vi "Text control 2 v6.5.vi"() -> ()   [LabVIEW 2016]
panel:
  in  "Tab Control":enum32{"Main", "Other parameters"}(tab)
  out "Line running":i32
  out "Total lines":i32
  out "Path":path=path "C:/users/rlp38/09Apr2009LTtesting/test2.txt"
  out "I vs Vg":cluster{"Y data in":dbl[], "X data in":dbl[]}[](graph)
  out "Is max":dbl format="%.2e"
  out "Id max":dbl format="%.2e"
  out "Ig max":dbl format="%.2e"
  out "Imax vs time":cluster{"Y data in":dbl[], "X data in":dbl[]}[](graph)
  out "Imin vs time":cluster{"Y data in":dbl[], "X data in":dbl[]}[](graph)
  out "I vs Vd":cluster{"Y data in":dbl[], "X data in":dbl[]}[](graph)
  in  "Script":string="#pulsedstressV d 0.03 20 0 0.5 0.0827 5\n#\n#itime m\n#gaterangemode a\n#drainrangemode a\n#pulsed on 0.05 0 0.02\n#transfer d -10 40 1 5 40 35\n#transfer d -10 40 1 5 40 35\n#transfer d -10 40 1 5 40 35\n#output d 0 40 20 0 40 1\n#\n#\n#sample 1 0.008 221 6 0.003\n#samplei 400e-6 200 6 0.002 0.1\n#vsu2pulse -10 4\n#\n#stressV 0.016 0.03 2e-4 0.1e-3 11\n#stressI 220e-7 0.08 15\n#transfer s -1 1 0.5 -0.005 0.005 0.005\n#output s 0 0 0 -0.008 0.008 0.002"
  out "Command running:":string
  out "Serial port data":string
  out "Elapsed Time":dbl caption="Elapsed Time (s)"
  in  "Time Units":u16(ring)=1 items=["Seconds", "Minutes", "Hours"]
  in  "Time Offset":dbl caption="Set Start Time (s)"
  in  "Reset":bool
  in  "Auto Reset":bool
  in  "integration time":u32(slide) max=2 step=1 scale=0.0..2.0
  out "Is on":dbl format="%.2e"
  out "Id on":dbl format="%.2e"
  out "Ig on":dbl format="%.2e"
  out "Ion vs time":cluster{"Y data in":dbl[], "X data in":dbl[]}[](graph)
  out "Ioff vs time":cluster{"Y data in":dbl[], "X data in":dbl[]}[](graph)
  out "Ig min":dbl format="%.2e"
  out "Id min":dbl format="%.2e"
  out "Is min":dbl format="%.2e"
  out "Is off":dbl format="%.2e"
  out "Id off":dbl format="%.2e"
  out "Ig off":dbl format="%.2e"
  in  "Integration time (long)":dbl=0.32 min=0.04 max=2.0 step=0.02 format="%.2f"
  in  "Integration time (short)":dbl=0.0019 min=8e-05 max=0.0019 step=8e-05 format="%^.0e"
  in  "Drain: Compliance":dbl=0.001 format="%.8f"
  in  "Gate: Compliance":dbl=0.001 format="%.8f"
  in  "Interrupt scan":bool
  in  "Interrupt program":bool
  in  "Plot output curve extrema vs time":bool
  in  "Plot transfer curve extrema vs time":bool
  in  "Gate Range\nmode":u16(ring) items=["Auto", "Limited", "Fixed"]
  in  "Gate Range":u8(slide)=6 max=11 scale=0.0..11.0
  in  "Source/Drain\nRange mode":u16(ring) items=["Auto", "Limited", "Fixed"]
  in  "Source/Drain Range":u8(slide)=6 max=11 scale=0.0..11.0
  in  "Panel Controls":T1={"Emergency Stop"=refnum, "TransGraph Max"=1e-05, "Text/Graph (text=false)"=TRUE} {"TransGraph Max" format="%.2e"}
  in  "Panel Controls 2":T2={"Emergency Stop"=refnum, "TransGraph Max"=1e-05, "Text/Graph (text=false)"=TRUE, "TransGraph Min"=1e-11} {"TransGraph Min" format="%.2e"; "TransGraph Max" format="%.2e"}
  out "error out":errorcluster
  in  "Delay before read (ms)":u32=1000
  in  "byte count":u32=64
  in  "Serial End Mode for Reads":u16(ring)=2 items=["None", "LastBit", "TermChar"]
  in  "Timeout (ms)":u32=10000
  in  "Enable Termination\nChar (T)":bool=TRUE
  in  "Termination char\n(0xA = '\\n' = LF)\n(0xD = '\\r' = CR)":u8=13 format="%.0x"
  in  "flow control":u16(ring) items=["None"=0, "XON/XOFF"=1, "RTS/CTS"=2, "DTR/DSR"=4]
  in  "stop bits":u16(ring)=10 items=["1.0"=10, "1.5"=15, "2.0"=20]
  in  "parity":u16(ring) items=["None", "Odd", "Even", "Mark", "Space"]
  in  "data bits":u16=8 min=5 max=8 step=1
  in  "VISA resource name":refnum<visa-resource-name>="COM6"
  in  "baud rate":u32=9600
  out "Timings Indicator":T3
  in  "Timings (overwritten by the Front Panel)":T4={"integration time"=0, "Short/Long integration time"=0.00064, "hold time (sec)"=0.0, "delay time (sec)"=0.0, "Step Time (0 disables)"=0.0, "sweep method"=0, "Pulse period"=0.005, "Base voltage"=0.0, "Pulse width"=0.0005} {"Pulse width" min=0.0005 max=0.1 step=0.0001 format="%.4f"; "Base voltage" format="%^.4e"; "Pulse period" min=0.005 max=1.0 step=0.0001 format="%.4f"; "sweep method" items=["Continuous", "Pulsed"]; "Step Time (0 disables)" format="%.2f"; "delay time (sec)" format="%.4f"; "hold time (sec)" format="%.4f"; "Short/Long integration time" format="%^.0e"; "integration time" scale=0.0..2.0}
  in  "SMU4":cluster{"on/off":bool, "Voltage":dbl} {"Voltage" min=-100.0 max=100.0 format="%.2f"}
  in  "Full Reset":bool
  in  "Standby":T5
  out "SMU4 Indicator":cluster{"on/off":bool, "Voltage":dbl} {"Voltage" min=-100.0 max=100.0 format="%.2f"}
  in  "Gate":T6={"Gate Start"=0.0, "Gate Stop"=2.0, "Gate Step (linear only)"=1.0, "Gate Compliance"=0.0001, "Gate PComp"=0.0, "Range mode"=0, "Range"=6} {"Range" max=11 scale=0.0..11.0; "Range mode" items=["Auto", "Limited", "Fixed"]; "Gate PComp" format="%^.2e"; "Gate Compliance" format="%^.2e"; "Gate Step (linear only)" format="%^.4e"; "Gate Stop" format="%^.4e"; "Gate Start" format="%^.4e"}
  in  "Drain 2":T7={"Drain Start"=0.0, "Drain Stop"=2.0, "Drain Compliance"=0.0001, "Drain Step"=1.0, "Drain PComp"=0.0, "Range mode"=0, "Range"=6} {"Range" max=11 scale=0.0..11.0; "Range mode" items=["Auto", "Limited", "Fixed"]; "Drain PComp" format="%^.2e"; "Drain Step" format="%^.4e"; "Drain Compliance" format="%^.2e"; "Drain Stop" format="%^.4e"; "Drain Start" format="%^.4e"}
  # "Time"
  # "Syntax:\nitime [s|m|l] time(sec): [s|m|l] determines the integration time setting (small|medium|long) and time sets the value.\nNOTE: The value of the integration time has to be within the range allowed by its category (s|m|l), otherwise, the closest value will be used. (e.g. if the category is set to short but the time value is very long, the actual value used will be the maximum short integration time.\nIntegration times:\n    Short: Default: 640 us. Range: 8E-5 - 1.92E-3 seconds.\n    Medium: Fixed at 1 NPL cycle (0.02 seconds).\n    Long: Default: 16 NPL cycles (0.32 seconds). Range: 2-100 NPL cycles (0.04 seconds - 2 seconds).\ngaterangemode [a|l|f]\ndrainrangemode [a|l|f]\npulsed [on|off] PulsePeriod(sec) PulseBaseVoltage PulseONWidth(sec)\nstandby [on l off]\nwait NumMilliseconds\nwait-min NumMinutes\n# texthere = comment\nSMU4 [ON|OFF] Voltage\ntransfer [s|d] VgStart VgStop VgStep VdStart VdStop VdStep\noutput [s|d] VgStart VgStop VgStep VdStart VdStop VdStep\nsample Vg Vd NumSamples Time(s) SampleInterval(s)\nsamplei Idg NumSamples Time(s) SampleInterval(s) VDGcompliance\n100 samples is approximately 13 seconds with medium integration\n# if in doubt use SampleInterval(s) = 0.004\nstressV VG VD IGcompliance IDcompliance Duration(sec)\nstressI IDG VDGcompliance Duration(sec)\nvsu2pulse Bias Duration(s)\npulsedstressV [s|d] VEstop VgON VgOFF Period(s) PulseONwidth(s) Vd\nsample-fpp Vg Vd NumSamples Time\nresample-fpp Vg Vd\ntransfer-fpp [s|d] VgStart VgStop VgStep VdStart VdStop VdStep\noutput-fpp [s|d] VgStart VgStop VgStep VdStart VdStop VdStep\nserial SerialPortCommand"
  # "1\n2\n3\n4\n5\n6\n7\n8\n9\n10\n11\n12\n13\n14\n15\n16\n17\n18\n19\n20"
  # "Serial port settings"
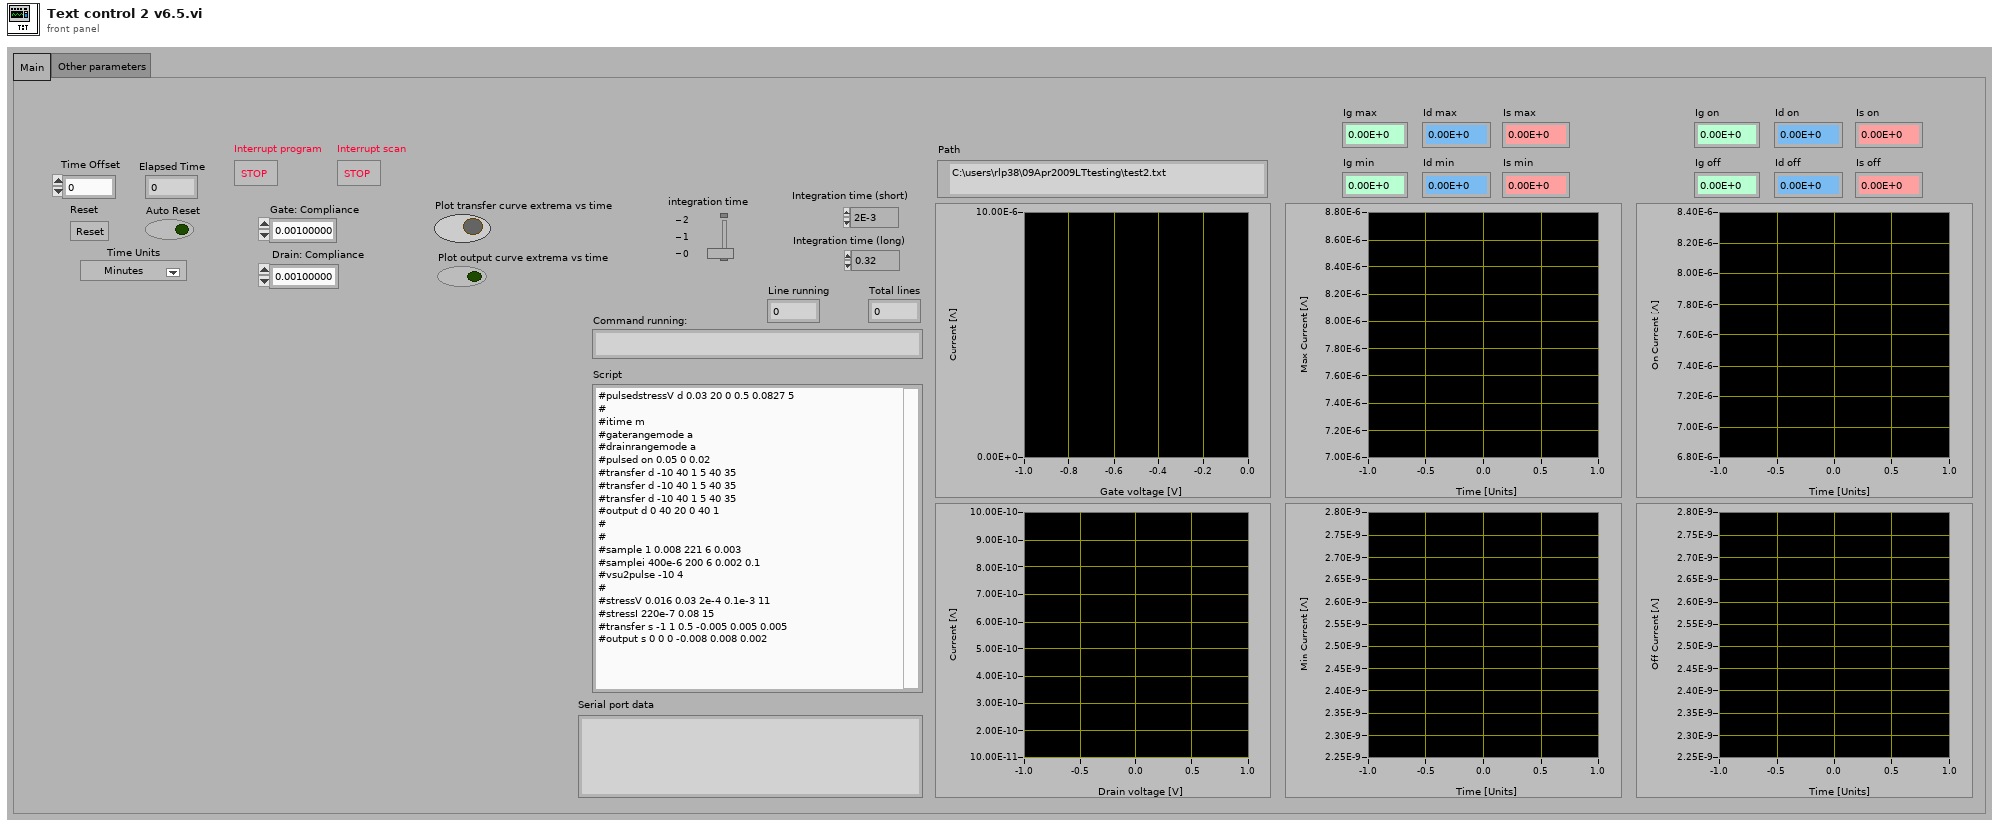
[diagram p1: front panel]
types:
  T1 = cluster{"Emergency Stop":refnum<vi>, "TransGraph Max":dbl, "Text/Graph (text=false)":bool}
  T2 = cluster{"Emergency Stop":refnum<vi>, "TransGraph Max":dbl, "Text/Graph (text=false)":bool, "TransGraph Min":dbl}
  T3 = cluster{"integration time (0:s, 1:m, 2:l)":u32, "Short/Long integration time":dbl, "hold time (sec)":dbl, "delay time (sec)":dbl, "Step Time (0 disables)":dbl, "sweep method":u16, "Pulse period":dbl, "Base voltage":dbl, "Pulse width":dbl}
  T4 = cluster{"integration time":u32, "Short/Long integration time":dbl, "hold time (sec)":dbl, "delay time (sec)":dbl, "Step Time (0 disables)":dbl, "sweep method":u16, "Pulse period":dbl, "Base voltage":dbl, "Pulse width":dbl}
  T5 = cluster{"Gate Standby":bool, "Drain Standby":bool}
  T6 = cluster{"Gate Start":dbl, "Gate Stop":dbl, "Gate Step (linear only)":dbl, "Gate Compliance":dbl, "Gate PComp":dbl, "Range mode":u16, "Range":u8}
  T7 = cluster{"Drain Start":dbl, "Drain Stop":dbl, "Drain Compliance":dbl, "Drain Step":dbl, "Drain PComp":dbl, "Range mode":u16, "Range":u8}
  T8 = enum16{"open", "replace", "create", "open or create", "replace or create", "replace or create with confirmation"}
  T9 = cluster{"V2 Start":dbl, "V2 Step":dbl, "Number of points":i32}
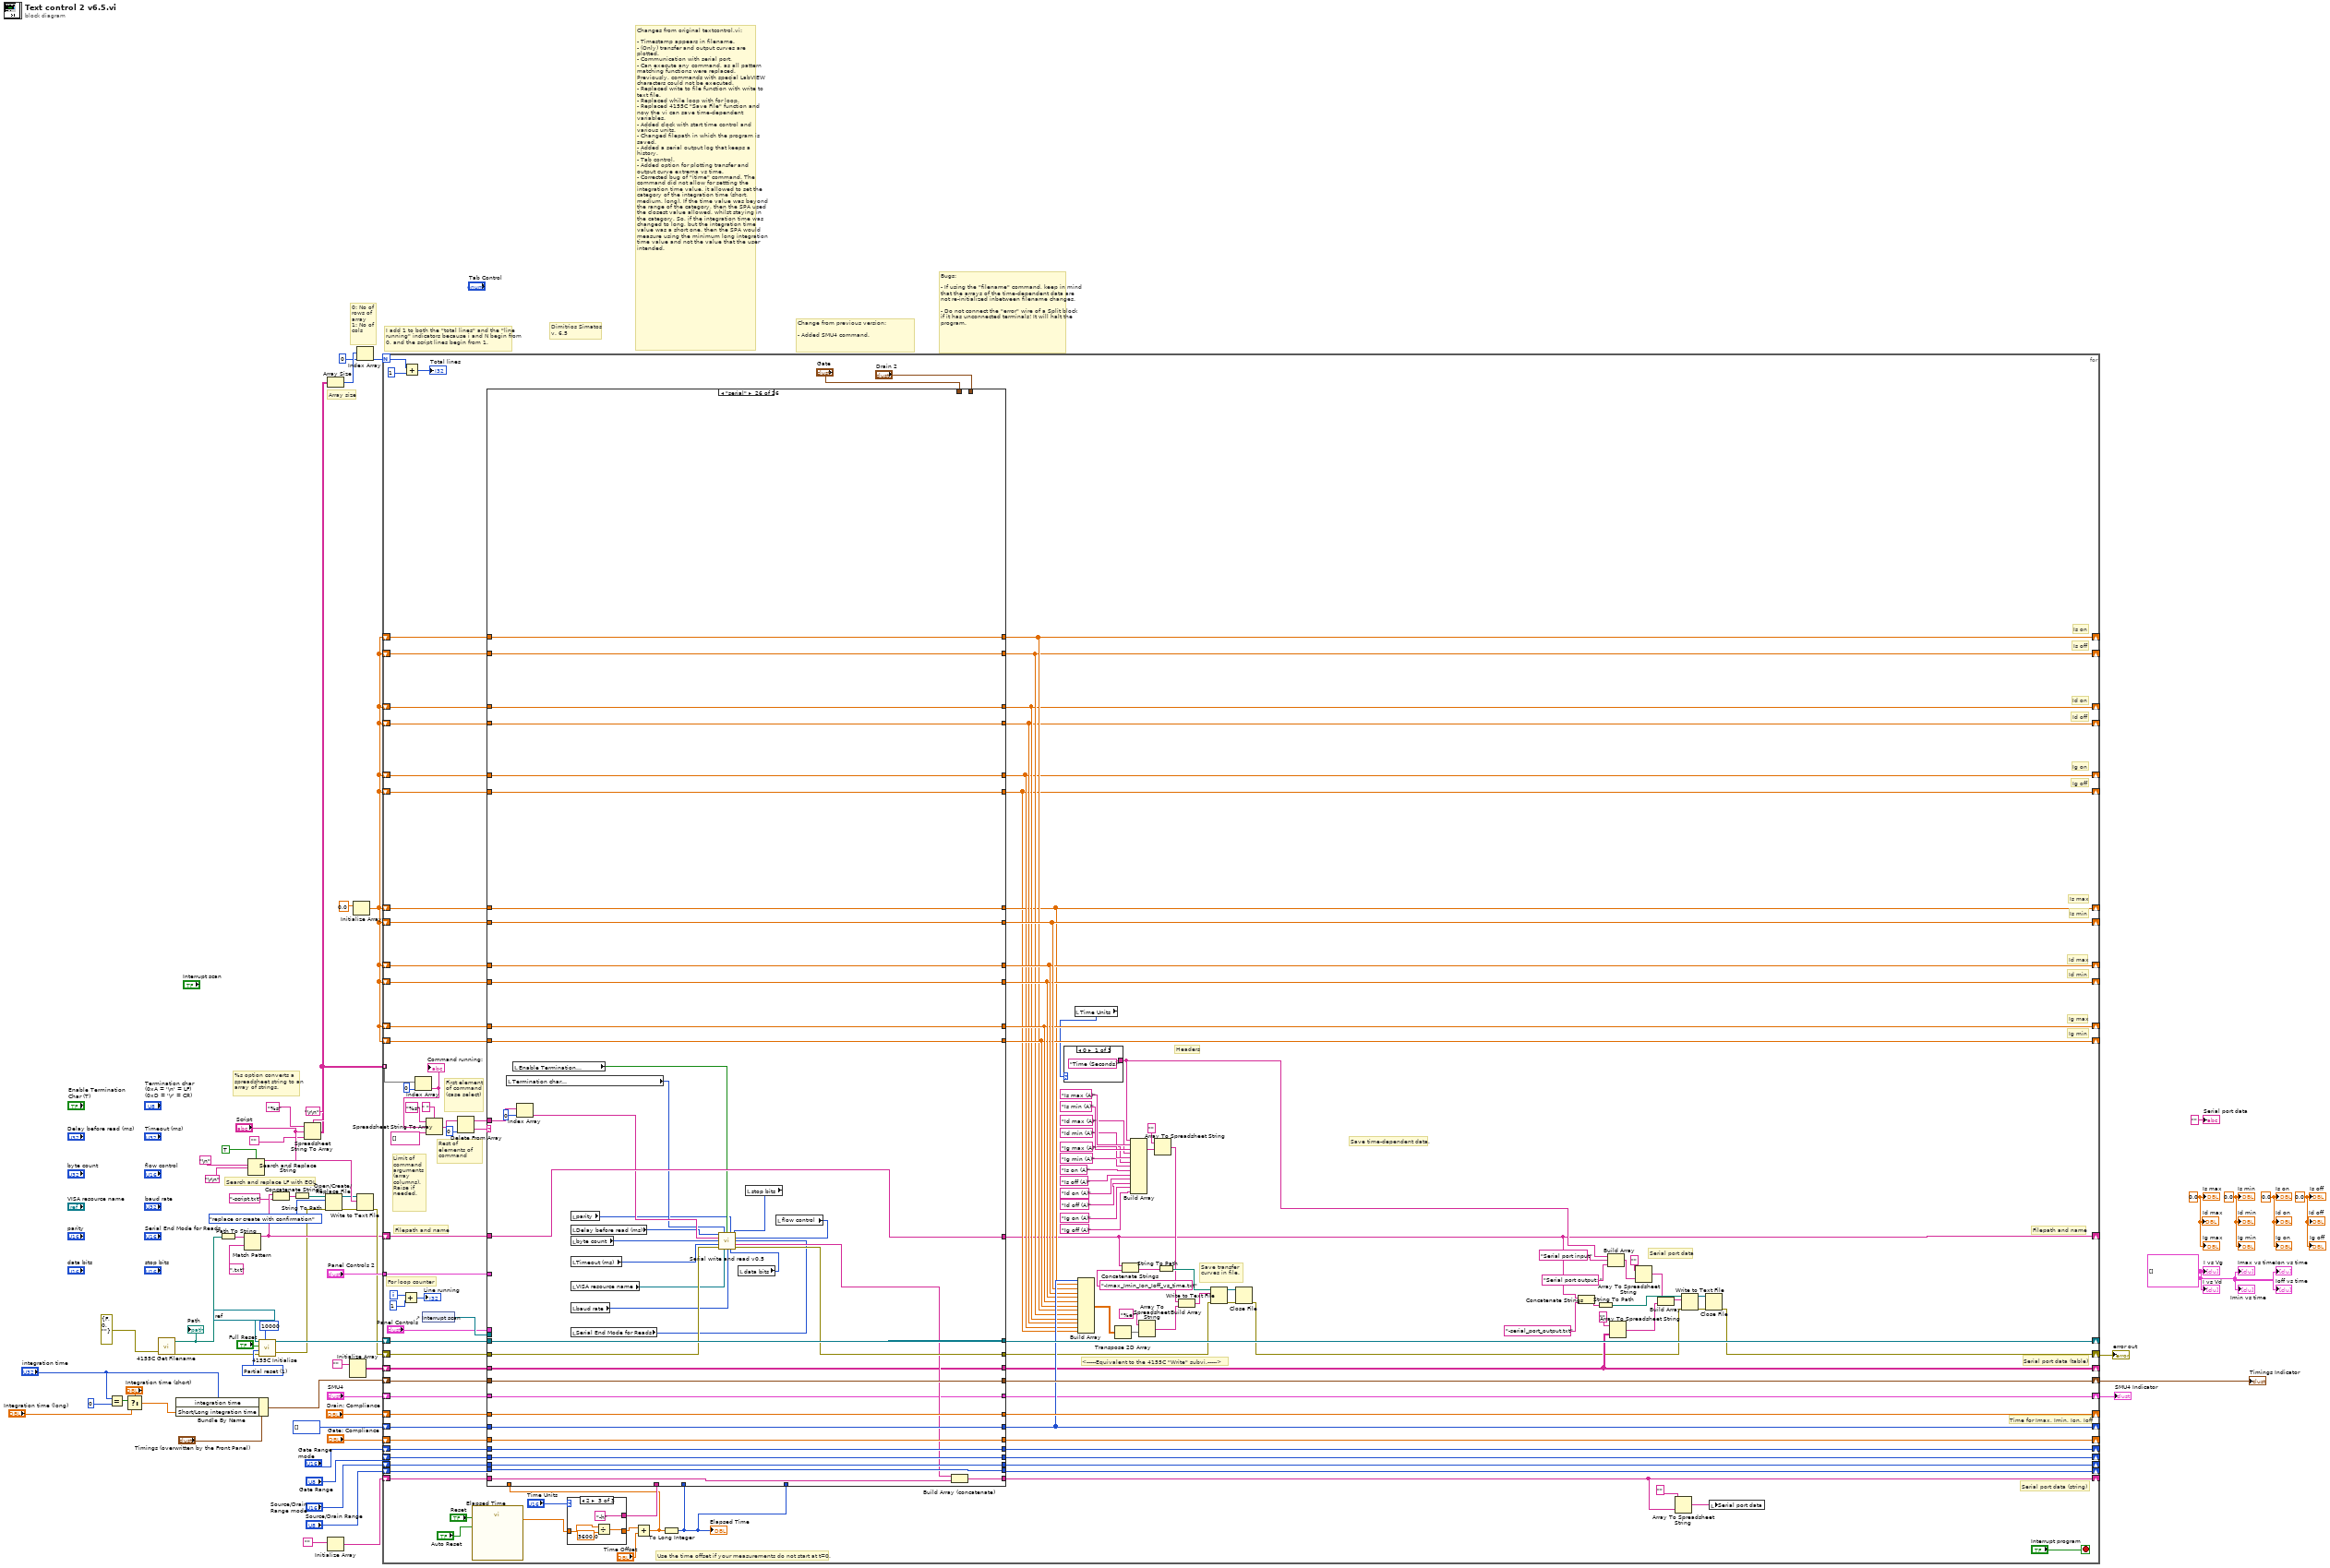
[diagram p0: block diagram]
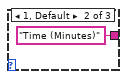
[diagram p2: hidden frame]
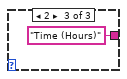
[diagram p3: hidden frame]
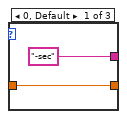
[diagram p4: hidden frame]
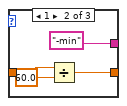
[diagram p5: hidden frame]
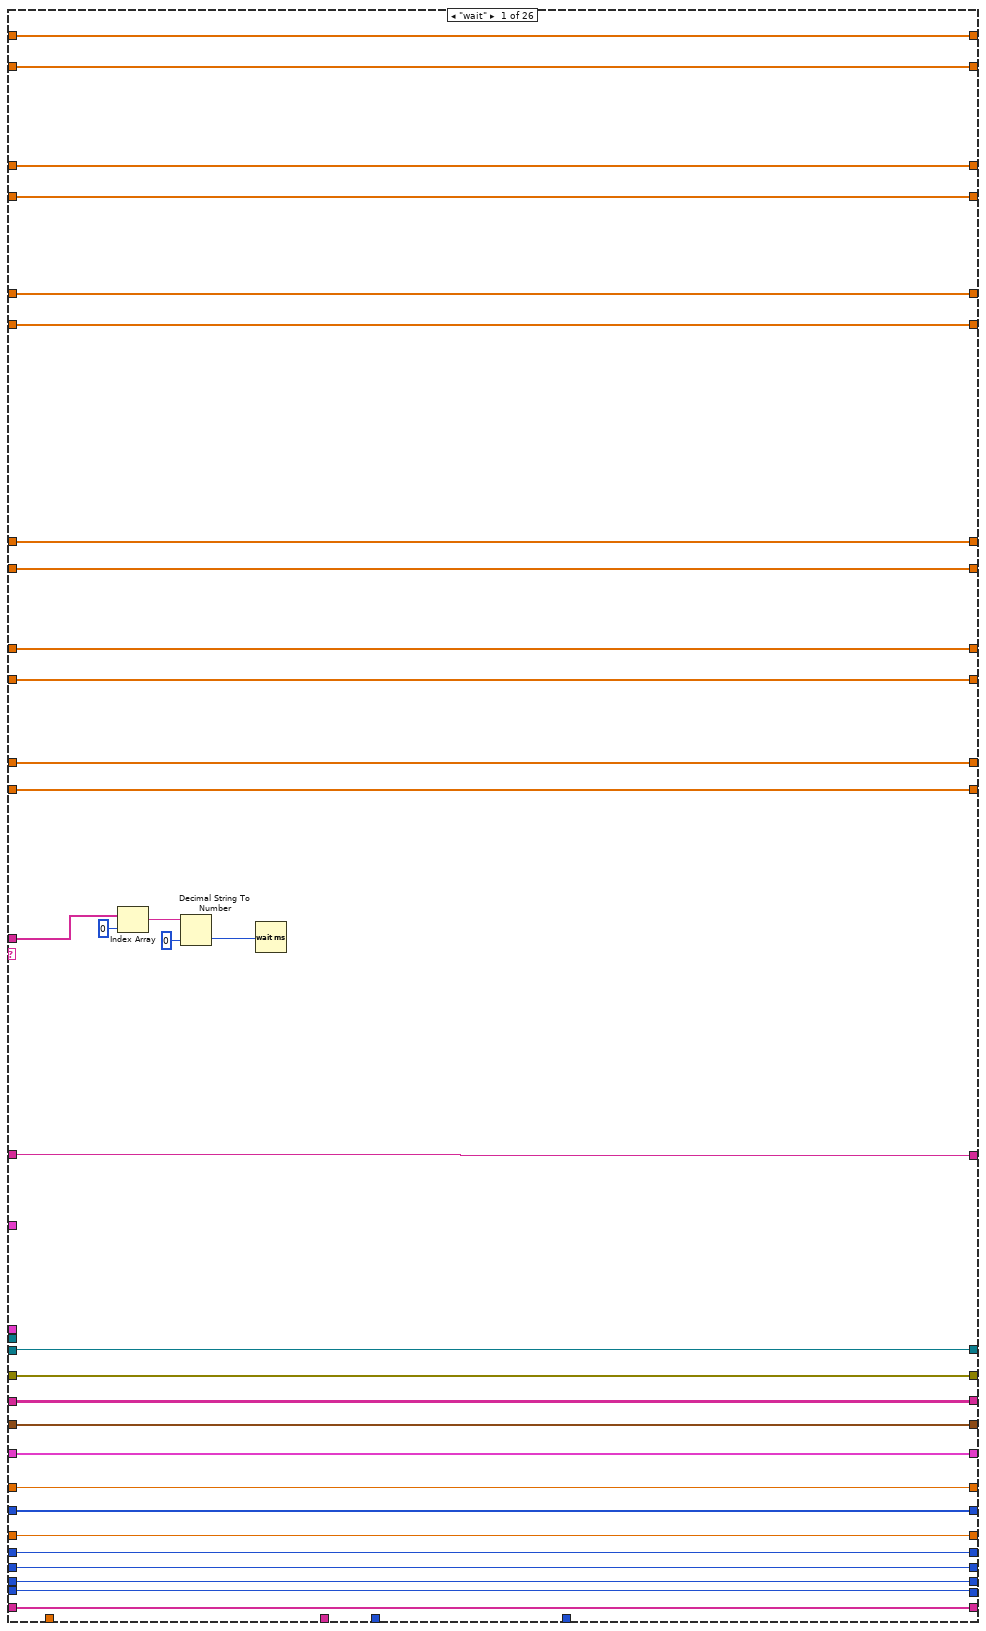
[diagram p6: hidden frame]
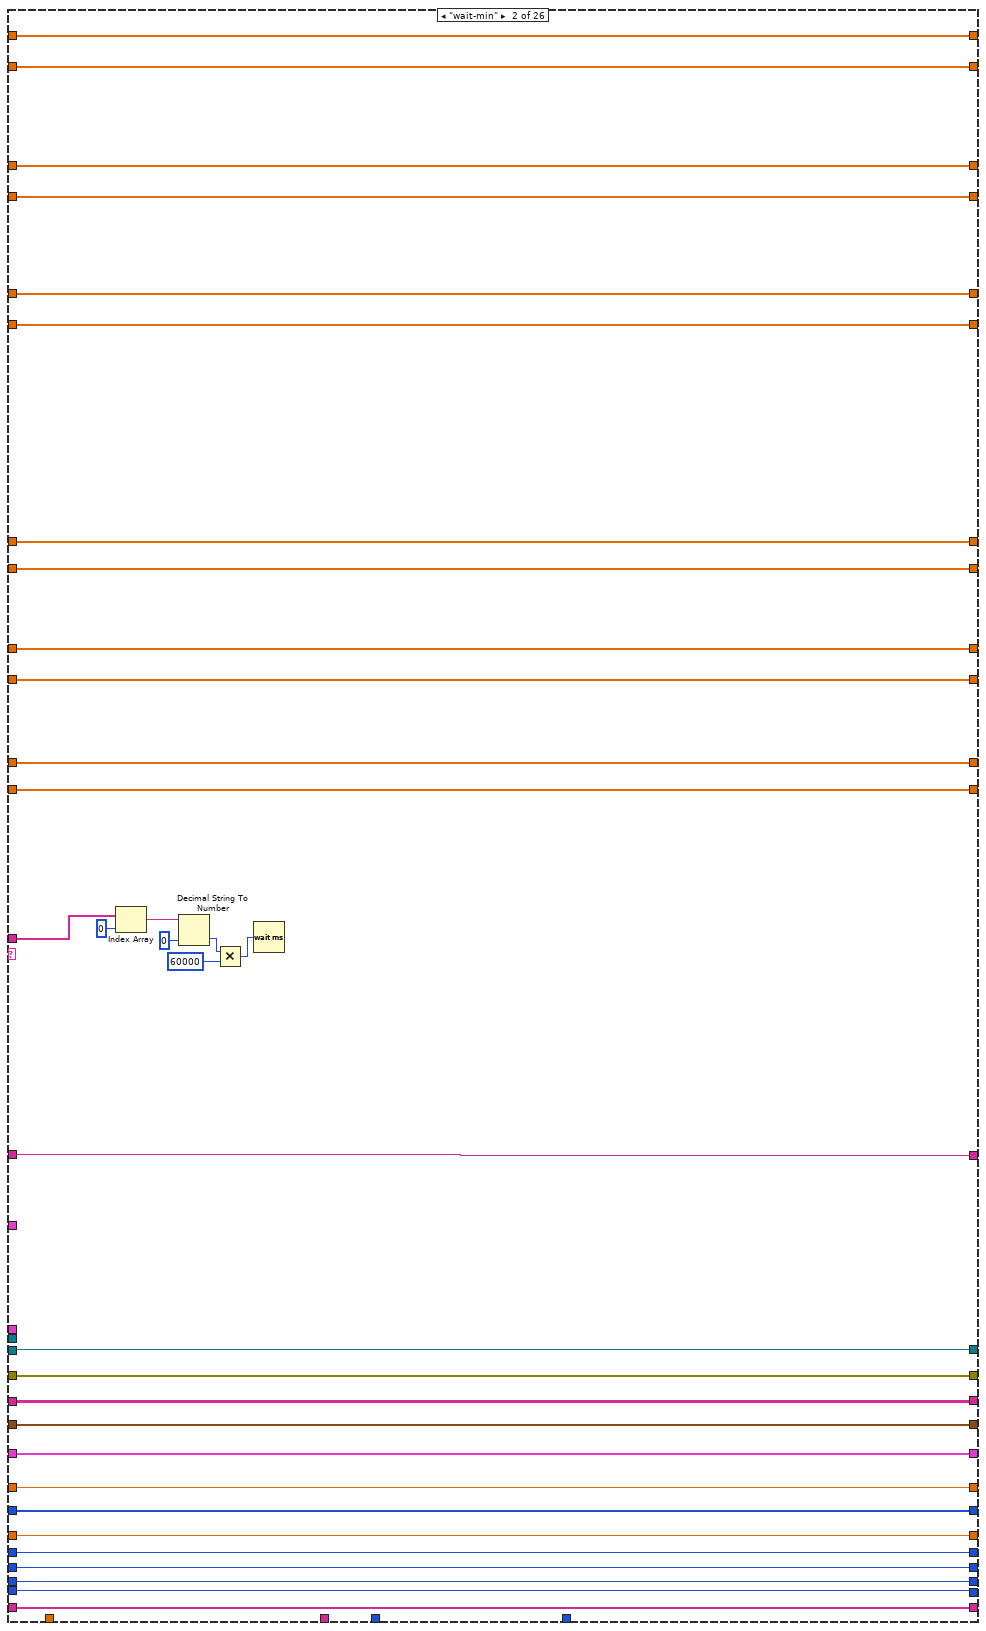
[diagram p7: hidden frame]
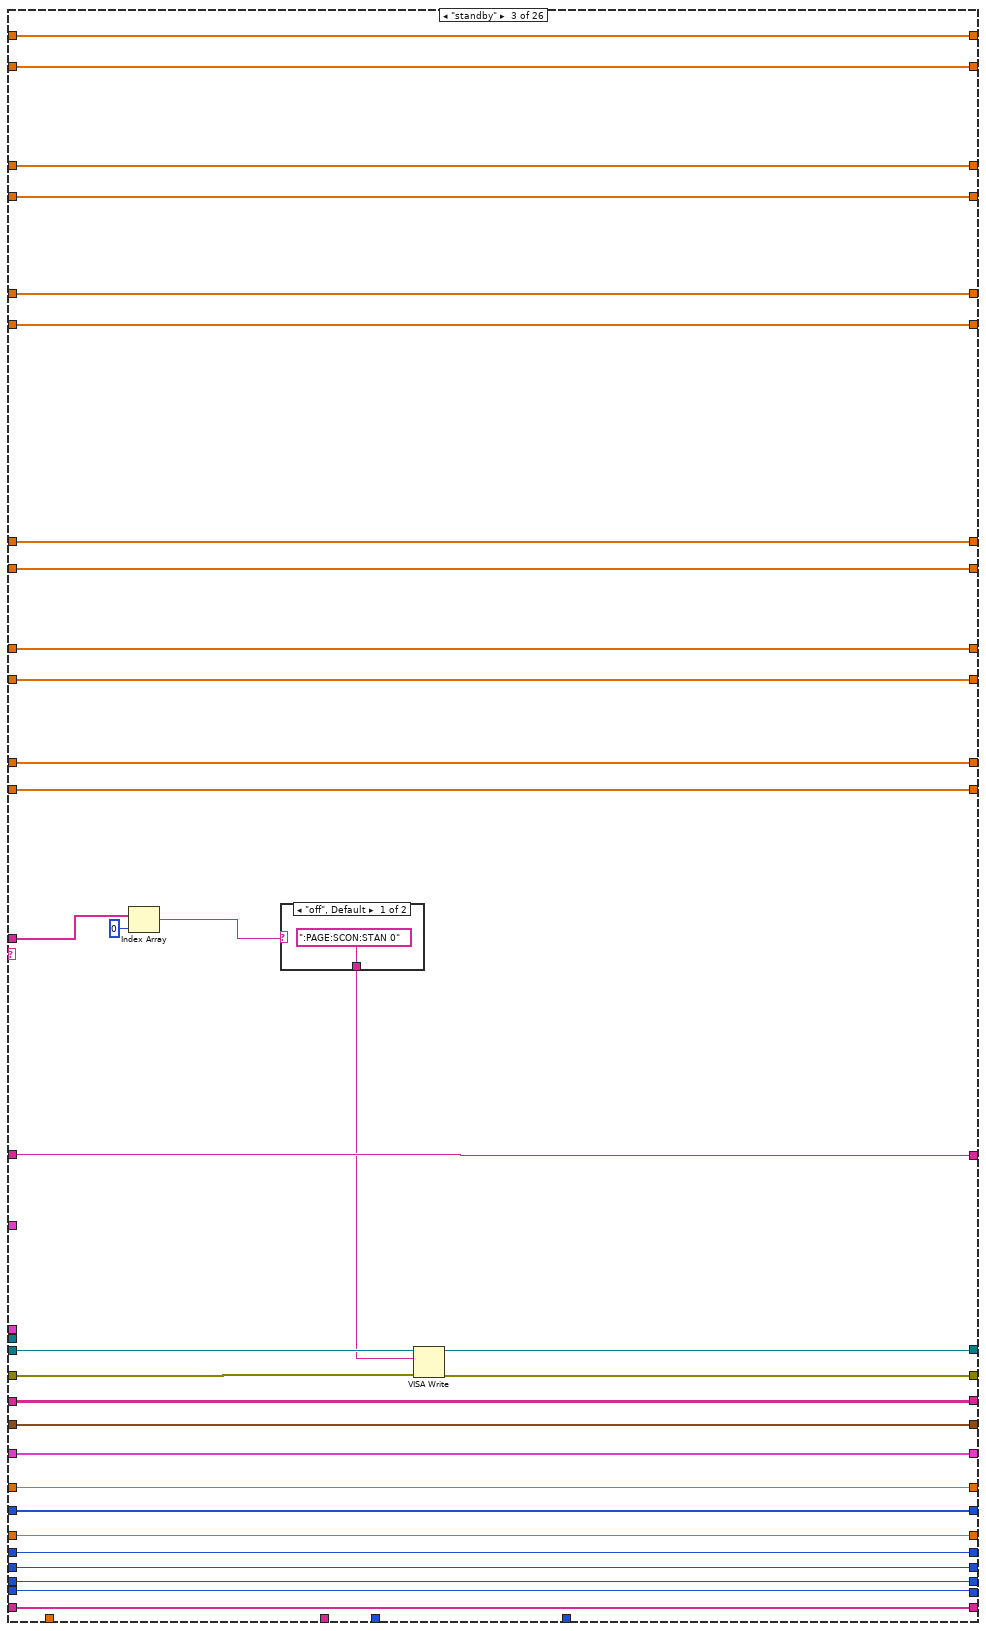
[diagram p8: hidden frame]
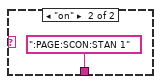
[diagram p9: hidden frame]
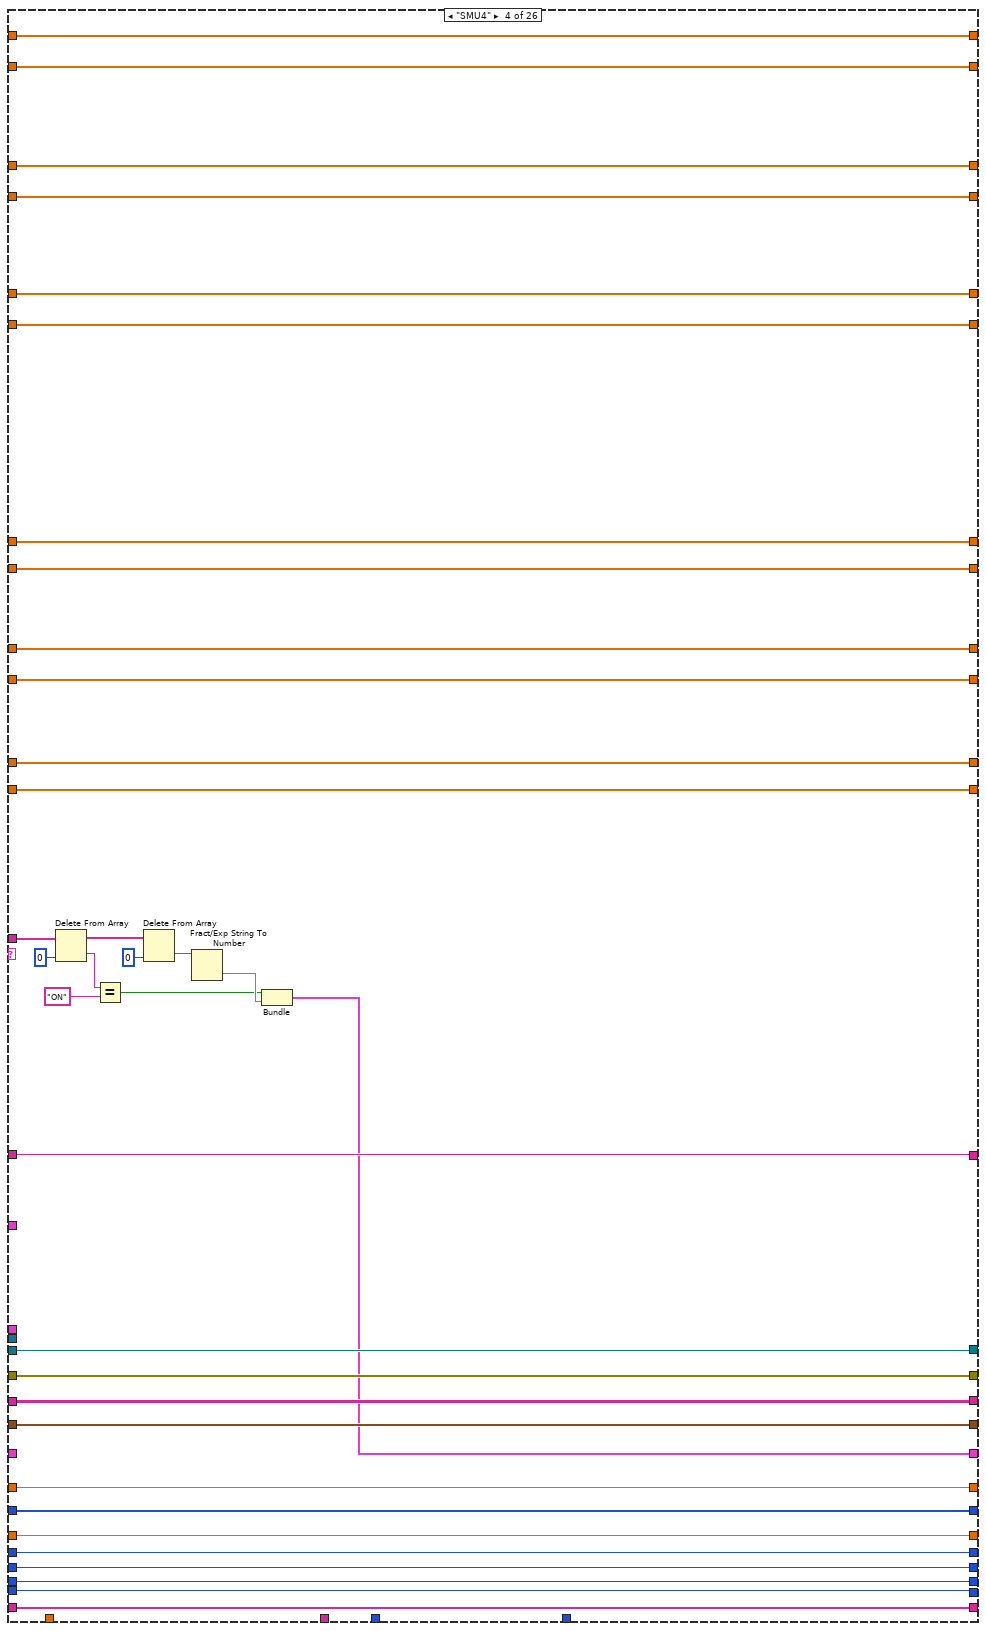
[diagram p10: hidden frame]
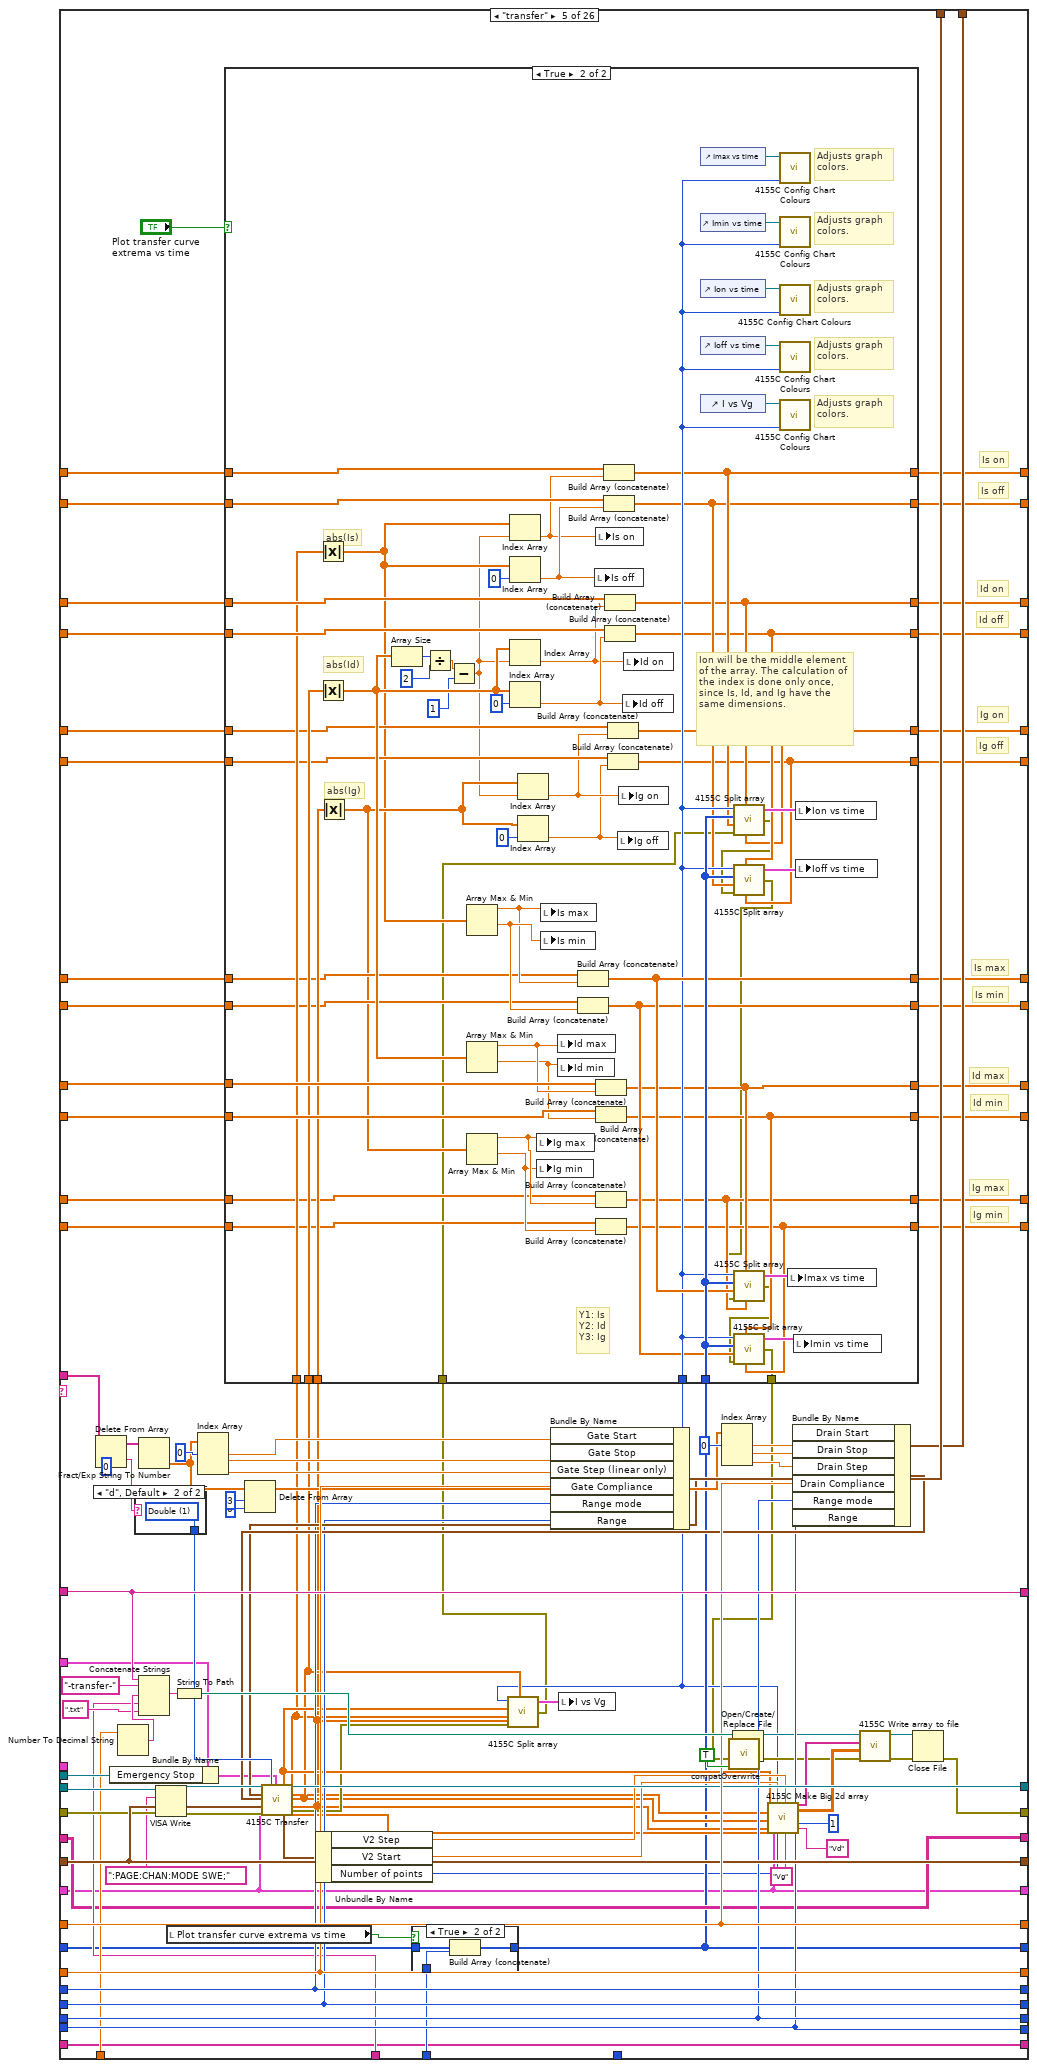
[diagram p11: hidden frame]
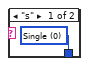
[diagram p14: hidden frame]
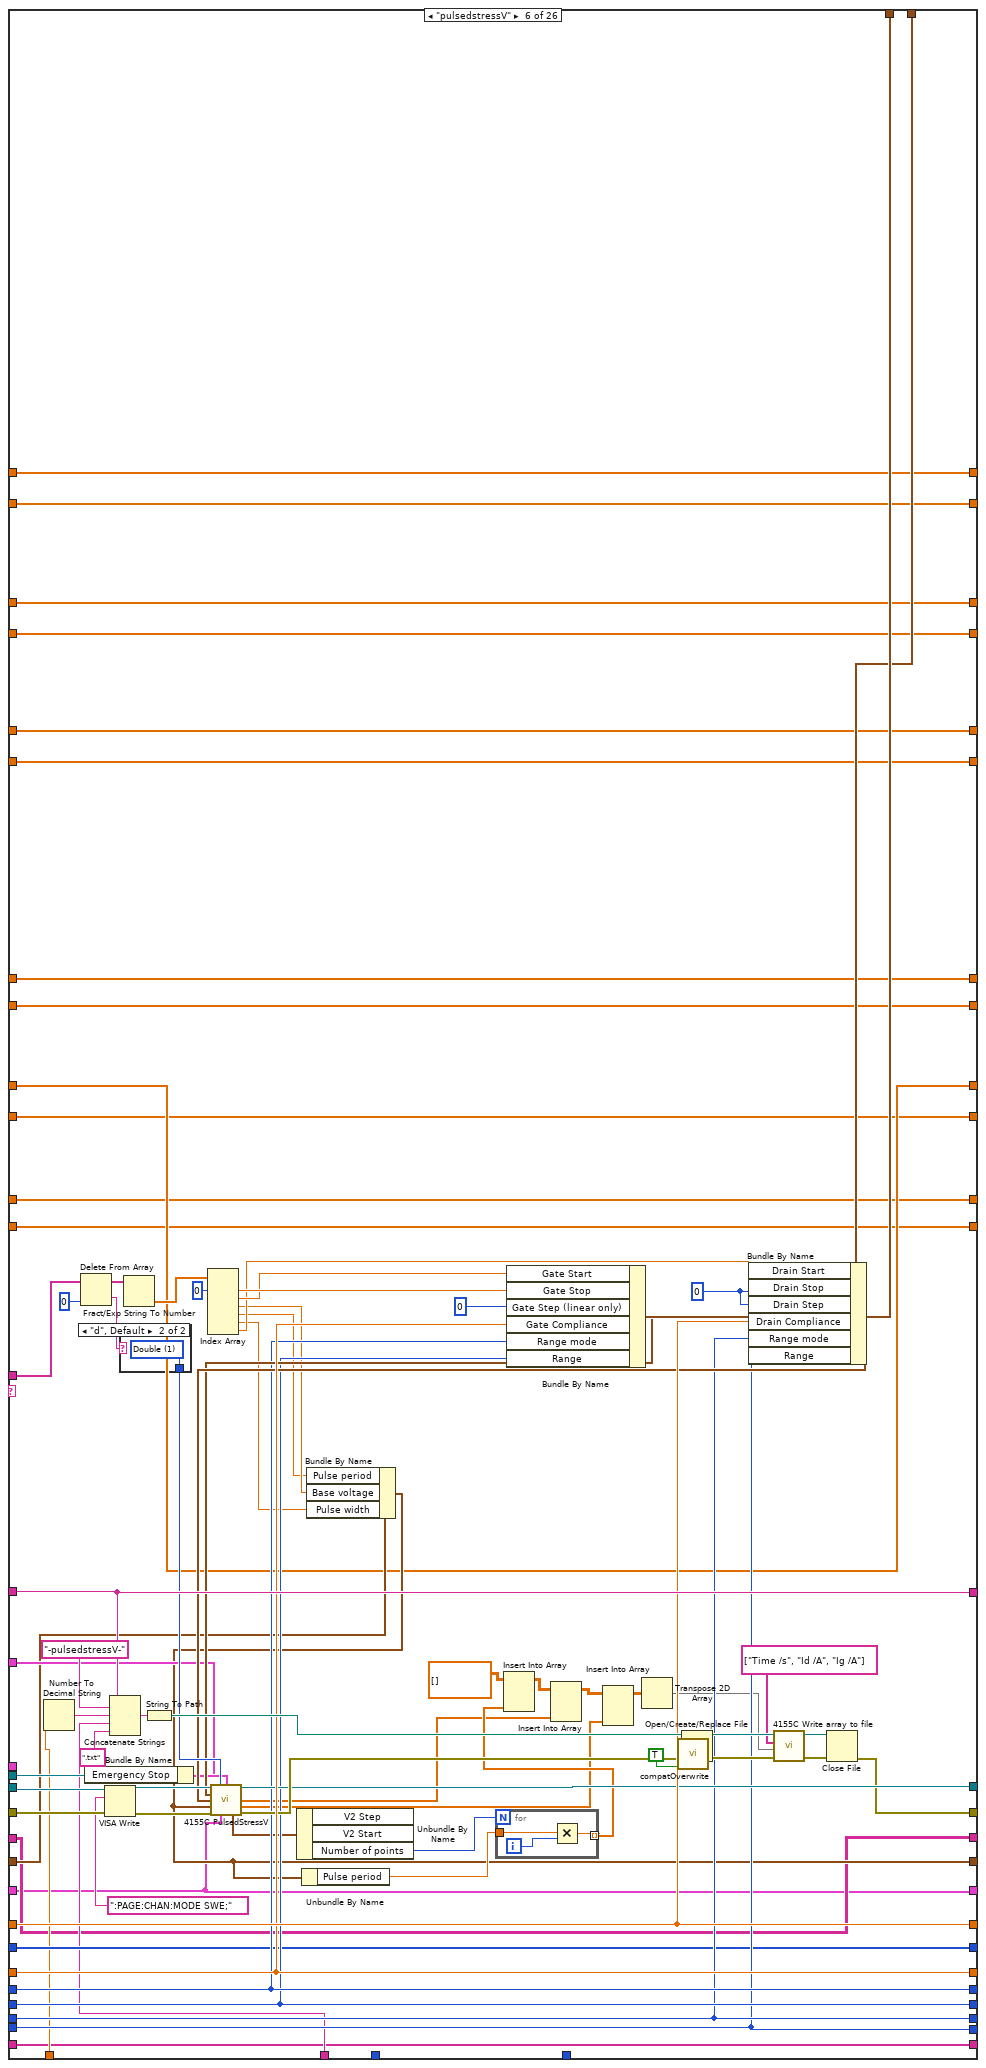
[diagram p15: hidden frame]
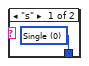
[diagram p16: hidden frame]
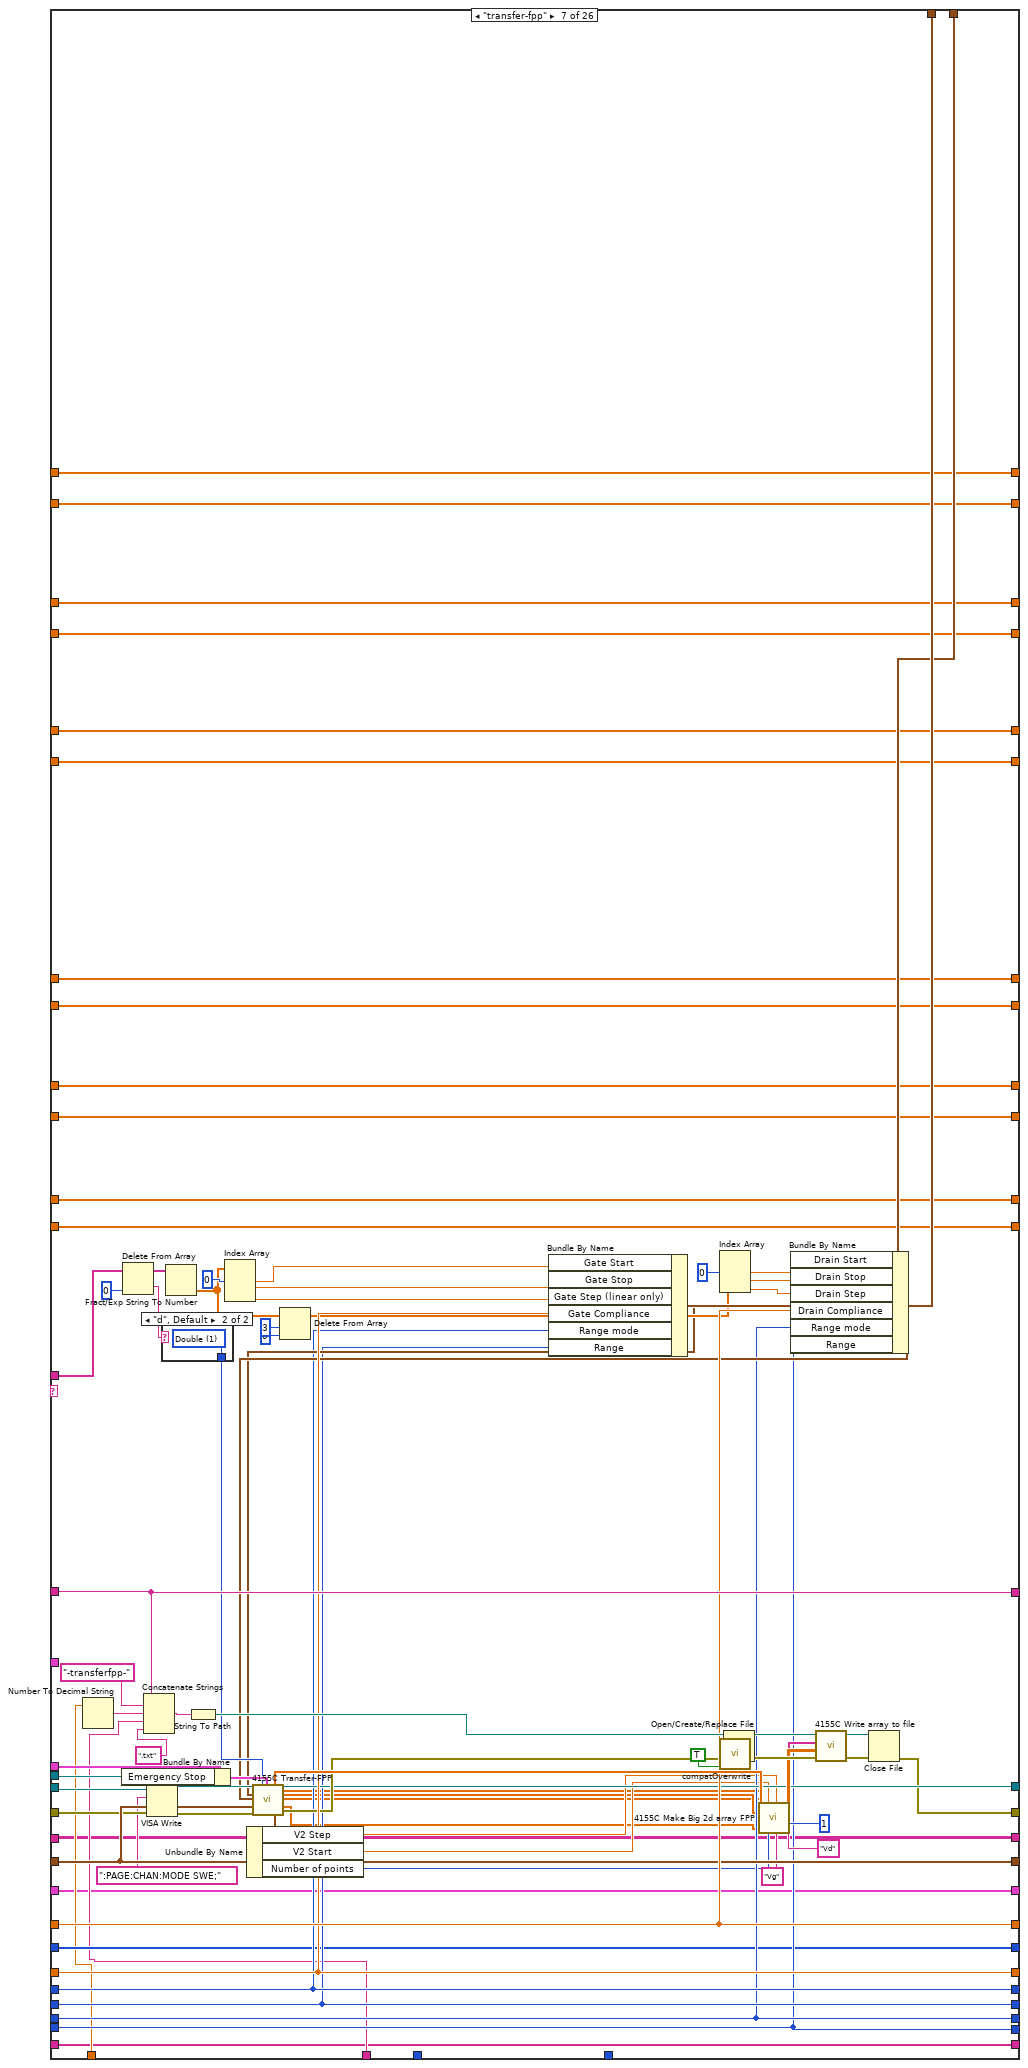
[diagram p17: hidden frame]
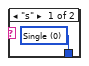
[diagram p18: hidden frame]
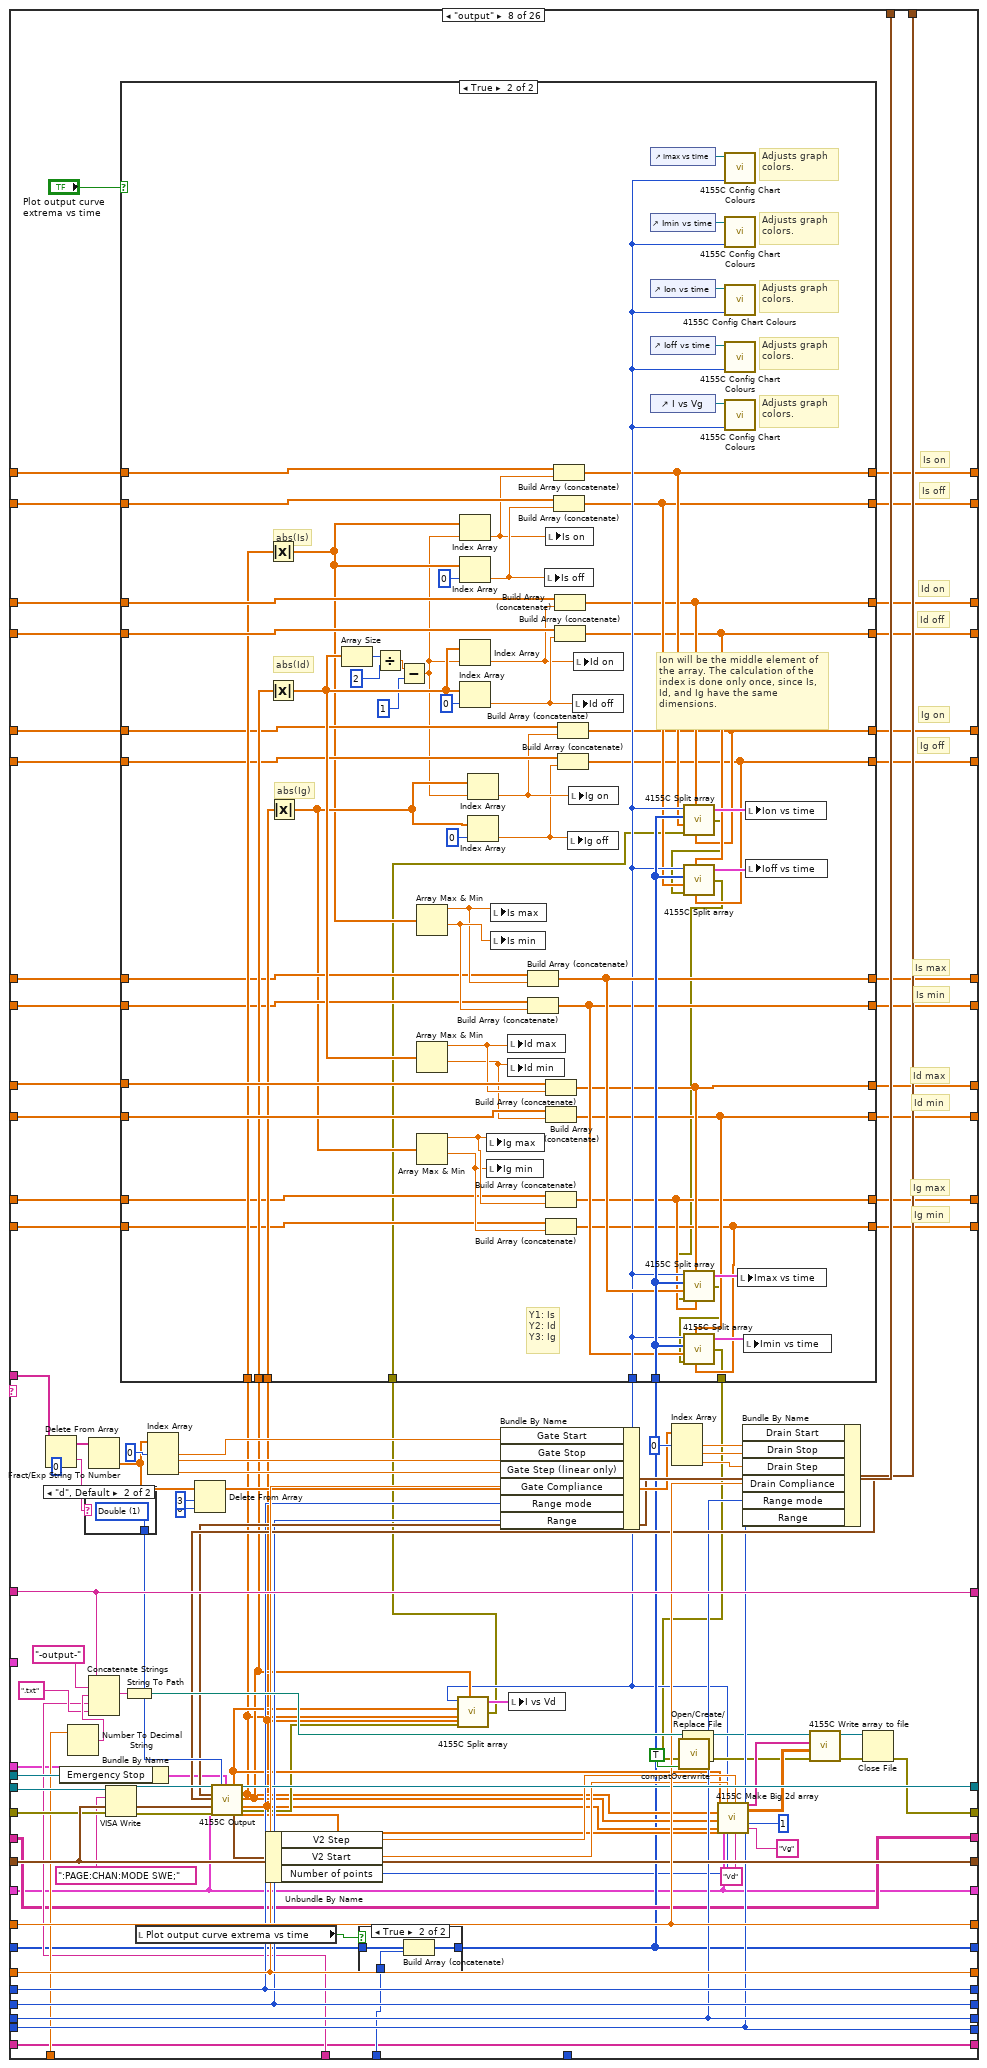
[diagram p19: hidden frame]
diagram:
  w8 = cluster{"Y data in":dbl[], "X data in":dbl[]}[] [] ("I vs Vg")
  w9 = 0.0 ("Is off")
  w10 = 0.0 ("Is on")
  w11 = 0.0 ("Is min")
  w12 = 0.0 ("Is max")
  w58 = u16 1 items=["Reset All", "Partial reset"] ("Type of reset")
  # "Change from previous version:\n\n- Added SMU4 command."
  # "I add 1 to both the \"total lines\" and the \"line running\" indicators because i and N begin from 0, and the script lines begin from 1."
  # "Bugs:\n\n- If using the \"filename\" command, keep in mind that the arrays of the time-dependent data are not re-initialized inbetween filename changes. \n\n- Do not connect the \"error\" wire of a Split block if it has unconnected terminals! It will halt the program."
  # "Array size"
  # "%s option converts a spreadsheet string to an array of strings."
  # "0: No of rows of array\n1: No of cols"
  # "Dimitrios Simatos\nv. 6.5"
  # "Changes from original textcontrol.vi:\n\n- Timestamp appears in filename.\n- (Only) transfer and output curves are plotted.\n- Communication with serial port.\n- Can execute any command, as all pattern matching functions were replaced. Previously, commands with special LabVIEW characters could not be executed.\n- Replaced write to file function with write to text file.\n- Replaced while loop with for loop.\n- Replaced 4155C \"Save File\" function and now the vi can save time-dependent variables.\n- Added clock with start time control and various units.\n- Changed filepath in which the program is saved.\n- Added a serial output log that keeps a history.\n- Tab control.\n- Added option for plotting transfer and output curve extrema vs time.\n- Corrected bug of \"itime\" command. The command did not allow for settting the integration time value, it allowed to set the category of the integration time (short, medium, long). If the time value was beyond the range of the category, then the SPA used the closest value allowed, whilst staying in the category. So, if the integration time was changed to long, but the integration time value was a short one, then the SPA would measure using the minimum long integration time value and not the value that the user intended."
  # "Search and replace LF with EOL"
  n1 = Equal?(x="integration time", y=u32 0) -> (x = y?=w59:bool)
  n2 = Select(t="Integration time (short)", s=w59, f="Integration time (long)") -> (s? t:f=w17:dbl)
  n3 = call "4155C Get Filename.vi"("error in (no error)"=errorcluster {"status"=FALSE, "code"=0, "source"=""}) -> ("error out"=w53:errorcluster, "path"=w28:path)  [unwired: 2 in, 1 out]
  "Path" <- w28
  n4 = Bundle By Name(cluster="Timings (overwritten by the Front Panel)", "integration time"="integration time", "Short/Long integration time"=w17) -> (w51:T4)
  n5 = Path To String(path=w28) -> (string=w29:string)
  n6 = Match Pattern(string=w29, regular expression=".txt") -> (before substring=w15:string)  [unwired: 1 in, 3 out]
  n7 = Search and Replace String(replace all?=TRUE ("replace all? (F)"), input string="Script", search string="\n", replace string="\r\n") -> (result string=w41:string)  [unwired: 4 in, 3 out]
  n8 = call "4155C Initialise.vi"("VISA resource name in"=refnum<visa-resource-name> "GPIB0::14::INSTR", "Reset"="Full Reset", "Type of reset"=w58, "error in (no error)"=w53, "VISA Timeout Value"=u32 10000) -> ("VISA Resource Name out"=w52:refnum<visa-resource-name>, "error out"=w6:errorcluster)
  n9 = Concatenate Strings(w15, "-script.txt" ("string")) -> (w16:string)
  n10 = String To Path(string=w16) -> (path=w4:path)
  n11 = Spreadsheet String To Array(delimiter (Tab)="\r\n", format string="%s", spreadsheet string="Script", array type (2D Dbl)="") -> (array=w32:string[][])
  n12 = Open/Create/Replace File(file path (use dialog)=w4, error in=w6, operation (0:open)=T8."replace or create with confirmation") -> (refnum out=w3:refnum<file>, error out=w5:errorcluster)  [unwired: 3 in, 1 out]
  n13 = Array Size(array=w32) -> (size(s)=w36:i32[])
  n14 = Initialize Array("") -> (w21:string[])  [unwired: 1 in]
  n15 = Initialize Array("") -> (w19:string[][])  [unwired: 2 in]
  n16 = Initialize Array(0.0 ("element")) -> (w23:dbl[])  [unwired: 1 in]
  n17 = Index Array(array=w36, index=0) -> (element=w34:i32)
  n18 = Write to Text File(file (use dialog)=w3, text=w41, error in=w5) -> (error out=w25:errorcluster)  [unwired: 1 in, 2 out]
  n19 = for {
    N: w34 -> [w132]
    shift-left: "Source/Drain Range" -> [w173]
    shift-right: [w169] -> _
    shift-left: "Source/Drain\nRange mode" -> [w174]
    shift-right: [w170] -> _
    shift-left: "Gate Range" -> [w175]
    shift-right: [w171] -> _
    shift-left: "Gate Range\nmode" -> [w176]
    shift-right: [w172] -> _
    shift-left: "Gate: Compliance" -> [w185]
    shift-right: [w181] -> _
    shift-left: "Drain: Compliance" -> [w186]
    shift-right: [w182] -> _
    shift-left: w51 -> [w187]
    shift-right: [w183] -> w18
    shift-left: w25 -> [w188]
    shift-right: [w68] -> w27
    shift-left: w52 -> [w189]
    shift-right: [w184] -> _
    shift-left: w15 -> [w190]
    shift-right: [w71] -> _
    tunnel: "Panel Controls 2" -> [w167]
    shift-right: [w83] -> _
    shift-left: w23 -> [w166]
    shift-right: [w119] -> _
    shift-left: i32[] [] -> [w162]
    tunnel: w32 -> [w161] mode=indexing
    shift-right: [w82] -> _
    shift-left: w23 -> [w138]
    shift-right: [w113] -> _
    shift-left: w21 -> [w124]
    shift-right: [w114] -> _
    shift-left: w19 -> [w116]
    shift-right: [w76] -> _
    shift-left: w23 -> [w104]
    shift-right: [w77] -> _
    shift-left: w23 -> [w103]
    shift-right: [w81] -> _
    shift-left: w23 -> [w92]
    shift-right: [w80] -> _
    shift-left: w23 -> [w91]
    shift-right: [w74] -> _
    shift-left: w23 -> [w90]
    shift-right: [w84] -> _
    shift-left: w23 -> [w89]
    shift-right: [w75] -> _
    shift-left: w23 -> [w88]
    shift-right: [w73] -> _
    shift-left: w23 -> [w87]
    shift-right: [w79] -> _
    shift-left: w23 -> [w86]
    shift-right: [w78] -> _
    shift-left: w23 -> [w85]
    shift-right: [w64] -> w1
    shift-left: "SMU4" -> [w168]
    i -> [w127]
    stop <- "Interrupt program" stop-if-true
    # "Is off"
    # "Is on"
    # "Ig off"
    # "Ig on"
    # "Is min"
    # "Is max"
    # "Ig min"
    # "Ig max"
    # "Id min"
    # "Id max"
    # "Id off"
    # "Id on"
    # "Filepath and name"
    # "Limit of command arguments (array columns). Raise if needed."
    # "Serial port data (string)"
    # "Serial port data (table)"
    # "Serial port data"
    # "For loop counter"
    # "<-----Equivalent to the 4155C \"Write\" subvi.----->"
    # "Headers"
    # "Save transfer curves in file."
    # "Filepath and name"
    # "Save time-dependent data."
    # "Use the time offset if your measurements do not start at t=0."
    # "Time for Imax, Imin, Ion, Ioff"
    # "Rest of elements of command"
    # "First element of command\n(case select)"
    n20 = Add(x=w127, y=1) -> (x+y=→"Line running":i32)
    n21 = Add(x=w132, y=1) -> (x+y=→"Total lines":i32)
    n22 = Index Array(array=w161, index=0 ("line index")) -> (element=w156:string)
    "Command running:" <- w156
    n23 = control-ref of="Interrupt scan"() -> (w180:refnum<vi>)
    n24 = Spreadsheet String To Array(delimiter (Tab)=" ", format string="%s", spreadsheet string=w156, array type (2D Dbl)=string[] []) -> (array=w154:string[])
    n25 = Delete From Array(array=w154, index=0) -> (deleted portion=w105:string, array with subset deleted=w153:string[])  [unwired: 1 in]
    n26 = call "Elapsed Time"("Reset"="Reset", "Auto Reset"="Auto Reset") -> ("Elapsed Time (s)"=w163:dbl)  [unwired: 10 in, 7 out]
    n27 = case shown="2" "Time Units" {
      tunnel: ["-sec" "-min" "-h"] -> w164
      tunnel: [w194 w198 w201] -> w134
      tunnel: w163 -> [w194 w197 w202]
      frame 0, Default {
      }
      frame 1 {
        n28 = Divide(x=w197, y=60.0) -> (x/y=w198:dbl)
      }
      frame 2 {
        n29 = Divide(x=w202, y=3600.0) -> (x/y=w201:dbl)
      }
    }
    n30 = Add(x=w134, y="Time Offset") -> (x+y=w133:dbl)
    n31 = To Long Integer(number=w133) -> (32bit integer=w118:i32)
    "Elapsed Time" <- w118
    n32 = case shown="\"serial\"" w105 {
      tunnel: w153 -> [w234 w267 w299 w311 w428 w535 w670 w785 w941 w969 w1038 w1079 w1118 w1153 w1181 _ _ w1327 w1402 _ w1495 w1553 w1609 w1693 w1769 w1803]
      tunnel: w190 -> [w229 w263 w297 w324 w435 w594 w678 w792 w949 w986 w1027 w1071 w1111 w1147 w1174 w1207 w1263 w1305 w1384 w1429 w1482 w1540 w1597 w1687 w1765 w1805]
      tunnel: w189 -> [w228 w262 w288 w323 w406 w579 w647 w763 w917 w987 w1028 w1072 w1112 w1148 w1175 w1212 w1265 w1333 w1408 w1433 w1501 w1559 w1615 w1699 w1723 w1809]
      tunnel: w188 -> [w227 w261 w287 w322 w405 w578 w646 w762 w914 w988 w1029 w1073 w1113 w1149 w1176 w1211 w1236 w1332 w1407 w1432 w1500 w1558 w1614 w1698 w1722 w1808]
      tunnel: w187 -> [w226 w260 w296 w320 w431 w555 w674 w788 w945 w996 w1037 w1070 w1110 w1146 w1173 w1210 w1260 w1296 w1376 w1438 w1475 w1533 w1590 w1686 w1764 w1810]
      tunnel: w186 -> [w225 w259 w295 w319 w433 w592 w676 w790 w947 w995 w1036 w1078 w1117 w1152 w1180 w1209 w1245 w1331 w1406 w1441 w1499 w1557 w1613 w1697 w1773 w1811]
      tunnel: w185 -> [w224 w258 w294 w317 w432 w591 w675 w789 w946 w994 w1035 w1077 w1116 w1151 w1179 w1208 w1246 w1306 w1385 w1440 w1483 w1541 w1598 w1688 w1766 w1813]
      tunnel: [w228 w262 w286 w323 w430 w589 w672 w787 w943 w987 w1028 w1072 w1112 w1148 w1175 w1212 w1265 w1297 w1358 w1431 w1476 w1534 w1591 w1639 w1725 w1809] -> w184
      tunnel: [w227 w261 w285 w322 w429 w588 w671 w786 w942 w988 w1029 w1073 w1113 w1149 w1176 w1211 w1235 w1307 w1359 w1430 w1484 w1542 w1599 w1638 w1724 w1807] -> w117
      tunnel: [w226 w260 w296 w320 w431 w551 w674 w788 w945 w989 w1030 w1070 w1110 w1146 w1173 w1210 w1260 w1296 w1376 w1438 w1475 w1533 w1590 w1686 w1764 w1810] -> w183
      tunnel: [w225 w259 w295 w319 w433 w592 w676 w790 w947 w995 w1036 w1078 w1117 w1152 w1180 w1209 w1245 w1331 w1406 w1441 w1499 w1557 w1613 w1697 w1773 w1811] -> w182
      tunnel: [w224 w258 w294 w317 w432 w591 w675 w789 w946 w994 w1035 w1077 w1116 w1151 w1179 w1208 w1246 w1306 w1385 w1440 w1483 w1541 w1598 w1688 w1766 w1813] -> w181
      tunnel: [w229 w263 w297 w324 w435 w594 w678 w792 w949 w986 w1027 w1071 w1111 w1147 w1174 w1207 w1263 w1305 w1384 w1429 w1482 w1540 w1597 w1687 w1765 w1805] -> w71
      tunnel: w180 -> [_ _ _ _ w437 w598 w683 w794 w953 _ _ _ _ _ _ _ _ w1302 w1381 _ w1481 w1539 w1596 w1659 w1741 _]
      tunnel: "Gate" -> [_ _ _ _ w415 w582 w657 w772 w928 _ _ _ _ _ _ _ _ _ _ _ _ _ _ _ _ _]
      tunnel: "Drain 2" -> [_ _ _ _ w414 w581 w656 w771 w927 _ _ _ _ _ _ _ _ _ _ _ _ _ _ _ _ _]
      tunnel: "Panel Controls" -> [_ _ _ _ _ _ w655 w698 w926 _ _ _ _ _ _ _ _ _ _ _ _ _ _ _ _ _]
      tunnel: w176 -> [w223 w257 w293 w316 w399 w572 w640 w756 w912 w993 w1034 _ w1109 w1145 w1172 w1206 w1247 w1292 w1372 w1434 w1471 w1529 w1586 w1682 w1760 w1814]
      tunnel: w175 -> [w222 w256 w292 w315 w398 w571 w639 w755 w911 w992 w1033 w1076 _ w1136 w1178 w1205 w1248 w1293 w1373 w1435 w1472 w1530 w1587 w1683 w1761 w1815]
      tunnel: w174 -> [w221 w255 w291 w314 w397 w570 w638 w754 w910 w991 w1032 w1075 w1115 w1150 _ w1204 w1249 w1294 w1374 w1436 w1473 w1531 w1588 w1684 w1762 w1816]
      tunnel: w173 -> [w220 w254 w290 w313 w396 w569 w637 w753 w913 w990 w1031 w1074 w1114 _ w1177 w1203 w1250 w1295 w1375 w1437 w1474 w1532 w1589 w1685 w1763 w1817]
      tunnel: [w223 w257 w293 w316 w399 w572 w640 w756 w912 w993 w1034 w1069 w1109 w1145 w1172 w1206 w1247 w1292 w1372 w1434 w1471 w1529 w1586 w1682 w1760 w1814] -> w172
      tunnel: [w222 w256 w292 w315 w398 w571 w639 w755 w911 w992 w1033 w1076 w1101 w1136 w1178 w1205 w1248 w1293 w1373 w1435 w1472 w1530 w1587 w1683 w1761 w1815] -> w171
      tunnel: [w221 w255 w291 w314 w397 w570 w638 w754 w910 w991 w1032 w1075 w1115 w1150 w1171 w1204 w1249 w1294 w1374 w1436 w1473 w1531 w1588 w1684 w1762 w1816] -> w170
      tunnel: [w220 w254 w290 w313 w396 w569 w637 w753 w913 w990 w1031 w1074 w1114 w1137 w1177 w1203 w1250 w1295 w1375 w1437 w1474 w1532 w1589 w1685 w1763 w1817] -> w169
      tunnel: w168 -> [w204 w235 w268 _ w337 w524 w609 w694 w881 w966 w1010 w1053 w1085 w1120 w1155 w1187 w1213 w1266 w1338 w1413 w1442 w1504 w1562 w1618 w1700 w1774]
      tunnel: w167 -> [_ _ _ _ w390 w566 _ _ _ _ _ _ _ _ _ _ _ _ _ _ _ _ _ _ _ _]
      tunnel: [w219 w250 w283 w328 w352 w543 w627 w710 w899 w985 w1025 w1068 w1100 w1135 w1170 w1202 w1231 w1284 w1342 w1428 w1460 w1522 w1580 w1636 w1718 w1806] -> w83
      tunnel: w166 -> [w219 w250 w283 w328 w387 w543 w627 w745 w899 w985 w1025 w1068 w1100 w1135 w1170 w1202 w1231 w1284 w1342 w1428 w1460 w1522 w1580 w1636 w1718 w1806]
      tunnel: w133 -> [_ _ _ _ w386 w540 w625 w744 w896 _ _ _ _ _ _ _ w1229 w1282 w1354 _ w1457 w1519 w1577 w1633 w1714 _]
      tunnel: w164 -> [_ _ _ _ w383 w539 w623 w741 w895 _ _ _ _ _ _ _ w1227 w1280 w1353 _ w1456 w1518 w1576 w1632 w1715 _]
      tunnel: w118 -> [_ _ _ _ w379 _ _ w737 _ _ _ _ _ _ _ _ _ _ _ _ _ _ _ _ _ _]
      tunnel: [w218 w249 w282 w318 w356 w542 w626 w714 w898 w984 w1024 w1067 w1099 w1134 w1169 w1201 w1230 w1283 w1356 w1427 w1459 w1521 w1579 w1635 w1717 w1812] -> w119
      tunnel: w162 -> [w218 w249 w282 w318 w382 w542 w626 w740 w898 w984 w1024 w1067 w1099 w1134 w1169 w1201 w1230 w1283 w1356 w1427 w1459 w1521 w1579 w1635 w1717 w1812]
      tunnel: [w217 w248 w281 w327 w351 w538 w622 w709 w894 w983 w1023 w1066 w1098 w1133 w1168 w1200 w1226 w1279 w1341 w1426 w1455 w1517 w1575 w1631 w1713 w1801] -> w82
      tunnel: w138 -> [w217 w248 w281 w327 w378 w538 w622 w736 w894 w983 w1023 w1066 w1098 w1133 w1168 w1200 w1226 w1279 w1341 w1426 w1455 w1517 w1575 w1631 w1713 w1801]
      tunnel: [w216 w247 w280 w312 w371 w537 w621 w729 w893 w982 w1022 w1065 w1097 w1132 w1167 w1199 w1225 w1278 w1352 w1425 w1454 w1516 w1574 w1630 w1712 w1800] -> w113
      tunnel: w124 -> [w216 w247 w280 w312 w371 w537 w621 w729 w893 w982 w1022 w1065 w1097 w1132 w1167 w1199 w1225 w1278 w1352 w1425 w1454 w1516 w1574 w1630 w1712 w1799]
      tunnel: w118 -> [_ _ _ _ _ _ _ _ _ _ _ _ _ _ _ _ _ _ _ _ _ _ _ _ _ _]
      tunnel: [w215 w246 w279 w321 w370 w536 w620 w728 w892 w981 w1021 w1064 w1096 w1131 w1166 w1198 w1224 w1277 w1351 w1424 w1453 w1515 w1573 w1629 w1711 w1785] -> w114
      tunnel: w116 -> [w215 w246 w279 w321 w370 w536 w620 w728 w892 w981 w1021 w1064 w1096 w1131 w1166 w1198 w1224 w1277 w1351 w1424 w1453 w1515 w1573 w1629 w1711 w1785]
      tunnel: [w213 w244 w277 w333 w345 w533 w618 w703 w890 w979 w1020 w1063 w1094 w1129 w1164 w1196 w1222 w1276 w1350 w1423 w1452 w1514 w1571 w1628 w1710 w1784] -> w76
      tunnel: w104 -> [w213 w244 w277 w333 w369 w533 w618 w727 w890 w979 w1020 w1063 w1094 w1129 w1164 w1196 w1222 w1276 w1350 w1423 w1452 w1514 w1571 w1628 w1710 w1784]
      tunnel: [w214 w245 w278 w334 w346 w534 w619 w704 w891 w980 w1019 w1062 w1095 w1130 w1165 w1197 w1223 w1275 w1349 w1422 w1451 w1513 w1572 w1627 w1709 w1783] -> w77
      tunnel: w103 -> [w214 w245 w278 w334 w368 w534 w619 w726 w891 w980 w1019 w1062 w1095 w1130 w1165 w1197 w1223 w1275 w1349 w1422 w1451 w1513 w1572 w1627 w1709 w1783]
      tunnel: [w206 w237 w270 w326 w350 w530 w616 w708 w888 w972 w1017 w1060 w1092 w1127 w1162 w1194 w1215 w1268 w1340 w1421 w1444 w1506 w1564 w1620 w1704 w1776] -> w81
      tunnel: w92 -> [w206 w237 w270 w326 w364 w530 w616 w722 w888 w972 w1017 w1060 w1092 w1127 w1162 w1194 w1215 w1268 w1340 w1421 w1444 w1506 w1564 w1620 w1704 w1776]
      tunnel: [w205 w236 w269 w325 w349 w531 w617 w707 w889 w971 w1018 w1061 w1093 w1128 w1163 w1195 w1214 w1267 w1339 w1420 w1443 w1505 w1563 w1619 w1703 w1775] -> w80
      tunnel: w91 -> [w205 w236 w269 w325 w363 w531 w617 w721 w889 w971 w1018 w1061 w1093 w1128 w1163 w1195 w1214 w1267 w1339 w1420 w1443 w1505 w1563 w1619 w1703 w1775]
      tunnel: [w208 w239 w272 w330 w355 w529 w614 w713 w886 w977 w1015 w1058 w1090 w1125 w1160 w1192 w1217 w1270 w1344 w1415 w1446 w1508 w1566 w1622 w1702 w1780] -> w74
      tunnel: w90 -> [w208 w239 w272 w330 w362 w529 w614 w720 w886 w977 w1015 w1058 w1090 w1125 w1160 w1192 w1217 w1270 w1344 w1415 w1446 w1508 w1566 w1622 w1702 w1780]
      tunnel: [w207 w238 w271 w329 w353 w532 w615 w711 w887 w978 w1016 w1059 w1091 w1126 w1161 w1193 w1216 w1269 w1343 w1414 w1445 w1507 w1565 w1621 w1701 w1779] -> w84
      tunnel: w89 -> [w207 w238 w271 w329 w361 w532 w615 w719 w887 w978 w1016 w1059 w1091 w1126 w1161 w1193 w1216 w1269 w1343 w1414 w1445 w1507 w1565 w1621 w1701 w1779]
      tunnel: [w210 w241 w274 w332 w344 w528 w612 w702 w884 w975 w1013 w1056 w1088 w1123 w1158 w1190 w1219 w1272 w1346 w1417 w1448 w1510 w1568 w1624 w1706 w1782] -> w75
      tunnel: w88 -> [w210 w241 w274 w332 w360 w528 w612 w718 w884 w975 w1013 w1056 w1088 w1123 w1158 w1190 w1219 w1272 w1346 w1417 w1448 w1510 w1568 w1624 w1706 w1782]
      tunnel: [w209 w240 w273 w331 w343 w527 w613 w701 w885 w976 w1014 w1057 w1089 w1124 w1159 w1191 w1218 w1271 w1345 w1416 w1447 w1509 w1567 w1623 w1705 w1781] -> w73
      tunnel: w87 -> [w209 w240 w273 w331 w359 w527 w613 w717 w885 w976 w1014 w1057 w1089 w1124 w1159 w1191 w1218 w1271 w1345 w1416 w1447 w1509 w1567 w1623 w1705 w1781]
      tunnel: [w212 w243 w276 w336 w348 w526 w610 w706 w882 w973 w1011 w1054 w1086 w1121 w1156 w1188 w1221 w1274 w1348 w1419 w1450 w1512 w1570 w1626 w1708 w1778] -> w79
      tunnel: w86 -> [w212 w243 w276 w336 w358 w526 w610 w716 w882 w973 w1011 w1054 w1086 w1121 w1156 w1188 w1221 w1274 w1348 w1419 w1450 w1512 w1570 w1626 w1708 w1778]
      tunnel: [w211 w242 w275 w335 w347 w525 w611 w705 w883 w974 w1012 w1055 w1087 w1122 w1157 w1189 w1220 w1273 w1347 w1418 w1449 w1511 w1569 w1625 w1707 w1777] -> w78
      tunnel: w85 -> [w211 w242 w275 w335 w357 w525 w611 w715 w883 w974 w1012 w1055 w1087 w1122 w1157 w1189 w1220 w1273 w1347 w1418 w1449 w1511 w1569 w1625 w1707 w1777]
      tunnel: [w204 w235 w268 w302 w337 w524 w609 w694 w881 w966 w1010 w1053 w1085 w1120 w1155 w1187 w1213 w1266 w1338 w1413 w1442 w1504 w1562 w1618 w1700 w1774] -> w64
      frame "wait" {
        n33 = Index Array(array=w234, index=0 ("Index")) -> (element=w232:string)
        n34 = Decimal String To Number(string=w232, default (0L)=u32 0) -> (number=w231:u32)  [unwired: 1 in, 1 out]
        n35 = Wait (ms)(milliseconds to wait=w231) -> ()  [unwired: 1 out]
      }
      frame "wait-min" {
        n36 = Index Array(array=w267, index=0 ("Index")) -> (element=w265:string)
        n37 = Decimal String To Number(string=w265, default (0L)=u32 0) -> (number=w253:u32)  [unwired: 1 in, 1 out]
        n38 = Multiply(x=w253, y=u32 60000) -> (x*y=w252:u32)
        n39 = Wait (ms)(milliseconds to wait=w252) -> ()  [unwired: 1 out]
      }
      frame "standby" {
        n40 = Index Array(array=w299, index=0 ("Index")) -> (element=w289:string)
        n41 = case shown="\"off\", Default" w289 {
          tunnel: [":PAGE:SCON:STAN 0" ":PAGE:SCON:STAN 1"] -> w284
          frame "off", Default {
          }
          frame "on" {
          }
        }
        n42 = VISA Write(VISA resource name=w288, write buffer=w284, error in (no error)=w287) -> (VISA resource name out=w286:refnum<visa-resource-name>, error out=w285:errorcluster)  [unwired: 1 out]
      }
      frame "SMU4" {
        n43 = Delete From Array(array=w311, index=0) -> (deleted portion=w305:string, array with subset deleted=w308:string[])  [unwired: 1 in]
        n44 = Equal?(x=w305, y="ON") -> (x = y?=w303:bool)
        n45 = Delete From Array(array=w308, index=0) -> (deleted portion=w307:string)  [unwired: 1 in, 1 out]
        n46 = Fract/Exp String To Number(string=w307) -> (number=w304:dbl)  [unwired: 3 in, 1 out]
        n47 = Bundle(w303, w304) -> (w302:cluster{bool, dbl})  [unwired: 1 in]
      }
      frame "transfer" {
        # "Is off"
        # "Is on"
        # "Ig off"
        # "Ig on"
        # "Is min"
        # "Is max"
        # "Ig min"
        # "Ig max"
        # "Id min"
        # "Id max"
        # "Id off"
        # "Id on"
        n48 = Delete From Array(array=w428, index=0 ("Index")) -> (deleted portion=w426:string, array with subset deleted=w425:string[])  [unwired: 1 in]
        n49 = Bundle By Name(cluster=w390, "Emergency Stop"=w437) -> (w391:T2)
        n50 = Number To Decimal String(number=w386) -> (decimal integer string=w385:string)  [unwired: 1 in]
        n51 = case shown="\"d\", Default" w426 {
          tunnel: [w522 w523] -> w424
          frame "s" {
            w522 = u16 0 items=["Single", "Double"] ("sweep mode")
          }
          frame "d", Default {
            w523 = u16 1 items=["Single", "Double"] ("sweep mode")
          }
        }
        n52 = Fract/Exp String To Number(string=w425) -> (number=w410:dbl[])  [unwired: 3 in, 1 out]
        n53 = Concatenate Strings(w435, "-transfer-" ("Prefix"), w385, w383, ".txt" ("Suffix (transfer)")) -> (w436:string)
        n54 = VISA Write(VISA resource name=w406, write buffer=":PAGE:CHAN:MODE SWE;" ("write buffer (\"\")"), error in (no error)=w405) -> (VISA resource name out=w403:refnum<visa-resource-name>, error out=w404:errorcluster)  [unwired: 1 out]
        n55 = local read "Plot transfer curve extrema vs time"() -> (w338:bool)
        n56 = String To Path(string=w436) -> (path=w434:path)
        n57 = Index Array(array=w410, index #1=0 ("Index")) -> (element #1=w423:dbl, element #2=w422:dbl, element #3=w421:dbl)  [unwired: 2 in]
        n58 = Delete From Array(array=w410, length=3 ("Length"), index=0 ("Index")) -> (array with subset deleted=w408:dbl[])  [unwired: 1 out]
        n59 = case shown="True" w338 {
          tunnel: w382 -> [w439 w442]
          tunnel: w379 -> [_ w441]
          tunnel: [w439 w440] -> w356
          frame False {
          }
          frame True {
            n60 = Build Array (concatenate)(w442, w441) -> (w440:i32[])
          }
        }
        n61 = Bundle By Name(cluster=w415, "Gate Start"=w423, "Gate Stop"=w422, "Gate Step (linear only)"=w421, "Gate Compliance"=w432, "Range mode"=w399, "Range"=w398) -> (w400:T6)
        n62 = Index Array(array=w408, index #1=0 ("Index")) -> (element #1=w418:dbl, element #2=w417:dbl, element #3=w416:dbl)  [unwired: 2 in]
        n63 = call <vilib>:"compatOverwrite.vi"("overwrite (F)"=TRUE) -> ("overwrite?"=w389:T8)
        n64 = Bundle By Name(cluster=w414, "Drain Start"=w418, "Drain Stop"=w417, "Drain Step"=w416, "Drain Compliance"=w433, "Range mode"=w397, "Range"=w396) -> (w401:T7)
        n65 = call "4155C Transfer.vi"("VISA resource name in"=w403, "Gate"=w400, "Drain"=w401, "Timings"=w431, "error in (no error)"=w404, "SMU4"=w337, "sweep mode"=w424, "Panel Controls"=w391) -> ("VG"=w388:dbl[], "Outparams"=w395:T9, "VISA Resource Name out"=w430:refnum<visa-resource-name>, "IS"=w366:dbl[], "ID"=w367:dbl[], "IG"=w365:dbl[], "error out"=w380:errorcluster, "SMU4"=w392:dbl[])  [unwired: 12 in]
        n66 = Unbundle By Name(w395) -> ("V2 Step"=w394:dbl, "V2 Start"=w393:dbl, "Number of points"=w354:i32)
        n67 = call "4155C Split array.vi"("Number of VAR2 steps"=w354, "Y2 data in"=w367, "X data in"=w388, "Y1 data in"=w366, "Y3 data in"=w365, "error in (no error)"=w380) -> ("Array of clusters"=w381:cluster{"Y data in":dbl[], "X data in":dbl[]}[], "error out"=w342:errorcluster)  [unwired: 1 in]
        n68 = case shown="True" "Plot transfer curve extrema vs time" {
          tunnel: w387 -> [w445 w521]
          tunnel: w378 -> [w446 w516]
          tunnel: w369 -> [w452 w512]
          tunnel: w368 -> [w453 w511]
          tunnel: w367 -> [_ w508]
          tunnel: w366 -> [_ w506]
          tunnel: w365 -> [_ w505]
          tunnel: w364 -> [w447 w501]
          tunnel: w363 -> [w449 w500]
          tunnel: w362 -> [w443 w497]
          tunnel: w361 -> [w444 w496]
          tunnel: w360 -> [w451 w493]
          tunnel: w359 -> [w450 w492]
          tunnel: w358 -> [w455 w489]
          tunnel: w357 -> [w454 w488]
          tunnel: w356 -> [_ w481]
          tunnel: [w443 w476] -> w355
          tunnel: w354 -> [_ w475]
          tunnel: [w444 w474] -> w353
          tunnel: [w445 w473] -> w352
          tunnel: [w446 w472] -> w351
          tunnel: [w447 w471] -> w350
          tunnel: [w449 w470] -> w349
          tunnel: [w455 w469] -> w348
          tunnel: [w454 w468] -> w347
          tunnel: [w453 w467] -> w346
          tunnel: [w452 w466] -> w345
          tunnel: [w451 w465] -> w344
          tunnel: [w450 w464] -> w343
          tunnel: w342 -> [w448 w463]
          tunnel: [w448 w459] -> w341
          frame False {
          }
          frame True {
            # "Adjusts graph colors."
            # "Adjusts graph colors."
            # "Ion will be the middle element of the array. The calculation of the index is done only once, since Is, Id, and Ig have the same dimensions."
            # "abs(Ig)"
            # "abs(Is)"
            # "Y1: Is\nY2: Id\nY3: Ig"
            # "abs(Id)"
            # "Adjusts graph colors."
            # "Adjusts graph colors."
            # "Adjusts graph colors."
            n69 = Absolute Value(x=w506) -> (abs(x)=w491:dbl[])
            n70 = Absolute Value(x=w508) -> (abs(x)=w507:dbl[])
            n71 = Absolute Value(x=w505) -> (abs(x)=w494:dbl[])
            n72 = Array Size(array=w507) -> (size(s)=w515:i32)
            n73 = Divide(x=w515, y=2) -> (x/y=w458:dbl)
            n74 = Subtract(x=w458, y=1) -> (x-y=w457:dbl)
            n75 = Array Max & Min(array=w491) -> (max value=w498:dbl, min value=w499:dbl)  [unwired: 2 out]
            n76 = Array Max & Min(array=w507) -> (max value=w520:dbl, min value=w504:dbl)  [unwired: 2 out]
            n77 = Array Max & Min(array=w494) -> (max value=w503:dbl, min value=w502:dbl)  [unwired: 2 out]
            n78 = Index Array(array=w491, index=w457) -> (element=w482:dbl)
            n79 = Index Array(array=w491, index=0) -> (element=w483:dbl)
            n80 = Index Array(array=w507, index=w457) -> (element=w484:dbl)
            n81 = Index Array(array=w507, index=0) -> (element=w485:dbl)
            n82 = Index Array(array=w494, index=w457) -> (element=w487:dbl)
            n83 = Index Array(array=w494, index=0) -> (element=w486:dbl)
            n84 = local write "Ig max"(w503) -> ()
            n85 = local write "Ig min"(w502) -> ()
            n86 = local write "Is max"(w498) -> ()
            n87 = local write "Is min"(w499) -> ()
            n88 = local write "Id max"(w520) -> ()
            n89 = local write "Id min"(w504) -> ()
            n90 = Build Array (concatenate)(w497, w498) -> (w476:dbl[])
            n91 = Build Array (concatenate)(w496, w499) -> (w474:dbl[])
            n92 = local write "Is off"(w483) -> ()
            n93 = local write "Is on"(w482) -> ()
            n94 = Build Array (concatenate)(w521, w520) -> (w473:dbl[])
            n95 = Build Array (concatenate)(w516, w504) -> (w472:dbl[])
            n96 = Build Array (concatenate)(w501, w503) -> (w471:dbl[])
            n97 = Build Array (concatenate)(w500, w502) -> (w470:dbl[])
            n98 = Build Array (concatenate)(w489, w482) -> (w469:dbl[])
            n99 = Build Array (concatenate)(w488, w483) -> (w468:dbl[])
            n100 = Build Array (concatenate)(w511, w484) -> (w467:dbl[])
            n101 = Build Array (concatenate)(w512, w485) -> (w466:dbl[])
            n102 = Build Array (concatenate)(w493, w487) -> (w465:dbl[])
            n103 = Build Array (concatenate)(w492, w486) -> (w464:dbl[])
            n104 = local write "Ig off"(w486) -> ()
            n105 = local write "Ig on"(w487) -> ()
            n106 = local write "Id off"(w485) -> ()
            n107 = local write "Id on"(w484) -> ()
            n108 = control-ref of="Imax vs time"() -> (w510:refnum<vi>)
            n109 = control-ref of="Imin vs time"() -> (w509:refnum<vi>)
            n110 = control-ref of="Ion vs time"() -> (w478:refnum<vi>)
            n111 = control-ref of="Ioff vs time"() -> (w477:refnum<vi>)
            n112 = control-ref of="I vs Vg"() -> (w519:refnum<vi>)
            n113 = call "4155C Split array.vi"("Number of VAR2 steps"=w475, "Y2 data in"=w467, "X data in"=w481, "Y1 data in"=w469, "Y3 data in"=w465, "error in (no error)"=w463) -> ("Array of clusters"=w479:cluster{"Y data in":dbl[], "X data in":dbl[]}[], "error out"=w462:errorcluster)  [unwired: 1 in]
            n114 = call "4155C Split array.vi"("Number of VAR2 steps"=w475, "Y2 data in"=w466, "X data in"=w481, "Y1 data in"=w468, "Y3 data in"=w464, "error in (no error)"=w462) -> ("Array of clusters"=w480:cluster{"Y data in":dbl[], "X data in":dbl[]}[], "error out"=w461:errorcluster)  [unwired: 1 in]
            n115 = call "4155C Split array.vi"("Number of VAR2 steps"=w475, "Y2 data in"=w473, "X data in"=w481, "Y1 data in"=w476, "Y3 data in"=w471, "error in (no error)"=w461) -> ("Array of clusters"=w518:cluster{"Y data in":dbl[], "X data in":dbl[]}[], "error out"=w460:errorcluster)  [unwired: 1 in]
            n116 = call "4155C Split array.vi"("Number of VAR2 steps"=w475, "Y2 data in"=w472, "X data in"=w481, "Y1 data in"=w474, "Y3 data in"=w470, "error in (no error)"=w460) -> ("Array of clusters"=w517:cluster{"Y data in":dbl[], "X data in":dbl[]}[], "error out"=w459:errorcluster)  [unwired: 1 in]
            n117 = call "4155C Config Chart Colours.vi"("Numeric"=w475, "XY Graph 2"=w510) -> ()  [unwired: 6 in]
            n118 = call "4155C Config Chart Colours.vi"("Numeric"=w475, "XY Graph 2"=w509) -> ()  [unwired: 6 in]
            n119 = call "4155C Config Chart Colours.vi"("Numeric"=w475, "XY Graph 2"=w478) -> ()  [unwired: 6 in]
            n120 = call "4155C Config Chart Colours.vi"("Numeric"=w475, "XY Graph 2"=w477) -> ()  [unwired: 6 in]
            n121 = call "4155C Config Chart Colours.vi"("Numeric"=w475, "XY Graph 2"=w519) -> ()  [unwired: 6 in]
            n122 = local write "Imax vs time"(w518) -> ()
            n123 = local write "Imin vs time"(w517) -> ()
            n124 = local write "Ion vs time"(w479) -> ()
            n125 = local write "Ioff vs time"(w480) -> ()
          }
        }
        n126 = local write "I vs Vg"(w381) -> ()
        n127 = Open/Create/Replace File(file path (use dialog)=w434, error in=w341, operation (0:open)=w389) -> (refnum out=w376:refnum<file>, error out=w374:errorcluster)  [unwired: 3 in, 1 out]
        n128 = call "4155C Make Big 2d array.vi"("1D Var1"=w388, "1d IS"=w366, "1d ID"=w367, "1d IG"=w365, "1d SMU4"=w392, "SMU4"=w337, "VAR2 START"=w393, "Number of VAR2 steps"=w354, "VAR2 STEP"=w394, "VAR1 Name"="Vg", "Decimal places in header"=i8 1, "VAR2 Name"="Vd") -> ("Header array"=w377:string[], "Data array"=w375:dbl[][])  [unwired: 14 in]
        n129 = call "4155C Write array to file.vi"("Byte Stream File Refnum"=w376, "Header"=w377, "Data Array"=w375, "error in (no error)"=w374) -> ("dup refnum"=w373:refnum<file>, "error out"=w372:errorcluster)  [unwired: 1 in]
        n130 = Close File(refnum=w373, error in=w372) -> (error out=w429:errorcluster)  [unwired: 1 out]
      }
      frame "pulsedstressV" {
        w549 = 0
        n131 = Number To Decimal String(number=w540) -> (decimal integer string=w595:string)  [unwired: 1 in]
        n132 = Delete From Array(array=w535, index=0 ("Index")) -> (deleted portion=w586:string, array with subset deleted=w585:string[])  [unwired: 1 in]
        n133 = Bundle By Name(cluster=w566, "Emergency Stop"=w598) -> (w567:T2)
        n134 = VISA Write(VISA resource name=w579, write buffer=":PAGE:CHAN:MODE SWE;" ("write buffer (\"\")"), error in (no error)=w578) -> (VISA resource name out=w576:refnum<visa-resource-name>, error out=w577:errorcluster)  [unwired: 1 out]
        n135 = Concatenate Strings(w594, "-pulsedstressV-" ("Substring"), w595, w539, ".txt" ("Substring")) -> (w597:string)
        n136 = case shown="\"d\", Default" w586 {
          tunnel: [w607 w608] -> w584
          frame "s" {
            w607 = u16 0 items=["Single", "Double"] ("sweep mode")
          }
          frame "d", Default {
            w608 = u16 1 items=["Single", "Double"] ("sweep mode")
          }
        }
        n137 = Fract/Exp String To Number(string=w585) -> (number=w580:dbl[])  [unwired: 3 in, 1 out]
        n138 = String To Path(string=w597) -> (path=w593:path)
        n139 = Index Array(array=w580, index #1=0 ("Index")) -> (element #1=w558:dbl, element #2=w557:dbl, element #3=w554:dbl, element #4=w553:dbl, element #5=w552:dbl, element #6=w556:dbl)  [unwired: 5 in]
        n140 = Bundle By Name(cluster=w555, "Pulse period"=w553, "Base voltage"=w554, "Pulse width"=w552) -> (w551:T4)
        n141 = Unbundle By Name(w551) -> ("Pulse period"=w559:dbl)
        n142 = Bundle By Name(cluster=w582, "Gate Start"=w557, "Gate Stop"=w558, "Gate Step (linear only)"=0, "Gate Compliance"=w591, "Range mode"=w572, "Range"=w571) -> (w573:T6)
        n143 = call <vilib>:"compatOverwrite.vi"("overwrite (F)"=TRUE) -> ("overwrite?"=w544:T8)
        n144 = Bundle By Name(cluster=w581, "Drain Start"=w556, "Drain Stop"=w549, "Drain Step"=w549, "Drain Compliance"=w592, "Range mode"=w570, "Range"=w569) -> (w574:T7)
        n145 = call "4155C PulsedStressV.vi"("VISA resource name in"=w576, "sweep mode"=w584, "Panel Controls"=w567, "Gate"=w573, "Drain"=w574, "Timings"=w551, "error in (no error)"=w577, "SMU4"=w524) -> ("VISA Resource Name out"=w589:refnum<visa-resource-name>, "ID"=w547:dbl[], "IG"=w545:dbl[], "Outparams"=w568:T9, "error out"=w590:errorcluster)  [unwired: 3 in]
        n146 = Unbundle By Name(w568) -> ("Number of points"=w546:i32)  [unwired: 2 out]
        n147 = for {
          N: w546 -> [_]
          tunnel: [w604] -> w548 mode=indexing
          tunnel: w559 -> [w606]
          i -> [w605]
          n148 = Multiply(x=w606, y=w605) -> (x*y=w604:dbl)
        }
        n149 = Insert Into Array(array=dbl[][] [] ("Input Array"), new element=w548) -> (w560:dbl[][])  [unwired: 2 in]
        n150 = Insert Into Array(array=w560, new element=w547) -> (w565:dbl[][])  [unwired: 2 in]
        n151 = Insert Into Array(array=w565, new element=w545) -> (w564:dbl[][])  [unwired: 2 in]
        n152 = Transpose 2D Array(2D array=w564) -> (transposed array=w563:dbl[][])
        n153 = Open/Create/Replace File(file path (use dialog)=w593, error in=w590, operation (0:open)=w544) -> (refnum out=w601:refnum<file>, error out=w602:errorcluster)  [unwired: 3 in, 1 out]
        n154 = call "4155C Write array to file.vi"("Byte Stream File Refnum"=w601, "Header"=string[] ["Time /s", "Id /A", "Ig /A"], "Data Array"=w563, "error in (no error)"=w602) -> ("dup refnum"=w599:refnum<file>, "error out"=w600:errorcluster)  [unwired: 1 in]
        n155 = Close File(refnum=w599, error in=w600) -> (error out=w588:errorcluster)  [unwired: 1 out]
      }
      frame "transfer-fpp" {
        n156 = Number To Decimal String(number=w625) -> (decimal integer string=w679:string)  [unwired: 1 in]
        n157 = Bundle By Name(cluster=w655, "Emergency Stop"=w683) -> (w691:T1)
        n158 = Delete From Array(array=w670, index=0 ("Index")) -> (deleted portion=w668:string, array with subset deleted=w667:string[])  [unwired: 1 in]
        n159 = Concatenate Strings(w678, "-transferfpp-" ("Substring"), w679, w623, ".txt" ("Substring")) -> (w681:string)
        n160 = VISA Write(VISA resource name=w647, write buffer=":PAGE:CHAN:MODE SWE;" ("write buffer (\"\")"), error in (no error)=w646) -> (VISA resource name out=w644:refnum<visa-resource-name>, error out=w645:errorcluster)  [unwired: 1 out]
        n161 = case shown="\"d\", Default" w668 {
          tunnel: [w692 w693] -> w666
          frame "s" {
            w692 = u16 0 items=["Single", "Double"] ("sweep mode")
          }
          frame "d", Default {
            w693 = u16 1 items=["Single", "Double"] ("sweep mode")
          }
        }
        n162 = Fract/Exp String To Number(string=w667) -> (number=w651:dbl[])  [unwired: 3 in, 1 out]
        n163 = String To Path(string=w681) -> (path=w677:path)
        n164 = Index Array(array=w651, index #1=0 ("Index")) -> (element #1=w665:dbl, element #2=w664:dbl, element #3=w663:dbl)  [unwired: 2 in]
        n165 = Delete From Array(array=w651, length=3 ("Length"), index=0 ("Index")) -> (array with subset deleted=w649:dbl[])  [unwired: 1 out]
        n166 = Bundle By Name(cluster=w657, "Gate Start"=w665, "Gate Stop"=w664, "Gate Step (linear only)"=w663, "Gate Compliance"=w675, "Range mode"=w640, "Range"=w639) -> (w641:T6)
        n167 = Index Array(array=w649, index #1=0 ("Index")) -> (element #1=w660:dbl, element #2=w659:dbl, element #3=w658:dbl)  [unwired: 2 in]
        n168 = call <vilib>:"compatOverwrite.vi"("overwrite (F)"=TRUE) -> ("overwrite?"=w628:T8)
        n169 = Bundle By Name(cluster=w656, "Drain Start"=w660, "Drain Stop"=w659, "Drain Step"=w658, "Drain Compliance"=w676, "Range mode"=w638, "Range"=w637) -> (w642:T7)
        n170 = call "4155C Transfer-FPP.vi"("VISA resource name in"=w644, "Gate"=w641, "Drain"=w642, "Timings"=w674, "error in (no error)"=w645, "sweep mode"=w666, "Panel Controls"=w691) -> ("VG"=w682:dbl[], "Outparams"=w636:T9, "VISA Resource Name out"=w672:refnum<visa-resource-name>, "Vprobe2"=w632:dbl[], "ID"=w631:dbl[], "IG"=w630:dbl[], "Vprobe1"=w629:dbl[], "error out"=w673:errorcluster)  [unwired: 13 in]
        n171 = Unbundle By Name(w636) -> ("V2 Step"=w635:dbl, "V2 Start"=w634:dbl, "Number of points"=w633:i32)
        n172 = Open/Create/Replace File(file path (use dialog)=w677, error in=w673, operation (0:open)=w628) -> (refnum out=w688:refnum<file>, error out=w689:errorcluster)  [unwired: 3 in, 1 out]
        n173 = call "4155C Make Big 2d array FPP.vi"("1D Var1"=w682, "1d ID"=w631, "1d Vp2"=w632, "1d IG"=w630, "1d Vp1"=w629, "VAR2 START"=w634, "Number of VAR2 steps"=w633, "VAR2 STEP"=w635, "VAR1 Name"="Vg", "Decimal places in header"=i8 1, "VAR2 Name"="Vd") -> ("Header array"=w684:string[], "Data array"=w685:dbl[][])  [unwired: 15 in]
        n174 = call "4155C Write array to file.vi"("Byte Stream File Refnum"=w688, "Header"=w684, "Data Array"=w685, "error in (no error)"=w689) -> ("dup refnum"=w686:refnum<file>, "error out"=w687:errorcluster)  [unwired: 1 in]
        n175 = Close File(refnum=w686, error in=w687) -> (error out=w671:errorcluster)  [unwired: 1 out]
      }
      frame "output" {
        # "Is off"
        # "Is on"
        # "Ig off"
        # "Ig on"
        # "Is min"
        # "Is max"
        # "Ig min"
        # "Ig max"
        # "Id min"
        # "Id max"
        # "Id off"
        # "Id on"
        n176 = Delete From Array(array=w785, index=0 ("Index")) -> (deleted portion=w783:string, array with subset deleted=w782:string[])  [unwired: 1 in]
        n177 = Bundle By Name(cluster=w698, "Emergency Stop"=w794) -> (w748:T1)
        n178 = Number To Decimal String(number=w744) -> (decimal integer string=w743:string)  [unwired: 1 in]
        n179 = case shown="\"d\", Default" w783 {
          tunnel: [w879 w880] -> w781
          frame "s" {
            w879 = u16 0 items=["Single", "Double"] ("sweep mode")
          }
          frame "d", Default {
            w880 = u16 1 items=["Single", "Double"] ("sweep mode")
          }
        }
        n180 = Fract/Exp String To Number(string=w782) -> (number=w767:dbl[])  [unwired: 3 in, 1 out]
        n181 = Concatenate Strings(w792, "-output-" ("Substring"), w743, w741, ".txt" ("Suffix (transfer)")) -> (w793:string)
        n182 = VISA Write(VISA resource name=w763, write buffer=":PAGE:CHAN:MODE SWE;" ("write buffer (\"\")"), error in (no error)=w762) -> (VISA resource name out=w760:refnum<visa-resource-name>, error out=w761:errorcluster)  [unwired: 1 out]
        n183 = String To Path(string=w793) -> (path=w791:path)
        n184 = local read "Plot output curve extrema vs time"() -> (w695:bool)
        n185 = Index Array(array=w767, index #1=0 ("Index")) -> (element #1=w780:dbl, element #2=w779:dbl, element #3=w778:dbl)  [unwired: 2 in]
        n186 = Delete From Array(array=w767, length=3 ("Length"), index=0 ("Index")) -> (array with subset deleted=w765:dbl[])  [unwired: 1 out]
        n187 = case shown="True" w695 {
          tunnel: w740 -> [w796 w799]
          tunnel: w737 -> [_ w798]
          tunnel: [w796 w797] -> w714
          frame False {
          }
          frame True {
            n188 = Build Array (concatenate)(w799, w798) -> (w797:i32[])
          }
        }
        n189 = Bundle By Name(cluster=w772, "Gate Start"=w780, "Gate Stop"=w779, "Gate Step (linear only)"=w778, "Gate Compliance"=w789, "Range mode"=w756, "Range"=w755) -> (w757:T6)
        n190 = Index Array(array=w765, index #1=0 ("Index")) -> (element #1=w775:dbl, element #2=w774:dbl, element #3=w773:dbl)  [unwired: 2 in]
        n191 = call <vilib>:"compatOverwrite.vi"("overwrite (F)"=TRUE) -> ("overwrite?"=w747:T8)
        n192 = Bundle By Name(cluster=w771, "Drain Start"=w775, "Drain Stop"=w774, "Drain Step"=w773, "Drain Compliance"=w790, "Range mode"=w754, "Range"=w753) -> (w758:T7)
        n193 = call "4155C Output.vi"("VISA resource name in"=w760, "Gate"=w757, "Drain"=w758, "Timings"=w788, "error in (no error)"=w761, "SMU4"=w694, "sweep mode"=w781, "Panel controls"=w748) -> ("VD"=w746:dbl[], "Outparams"=w752:T9, "VISA Resource Name out"=w787:refnum<visa-resource-name>, "IS"=w724:dbl[], "ID"=w725:dbl[], "IG"=w723:dbl[], "error out"=w738:errorcluster, "SMU4"=w749:dbl[])  [unwired: 12 in]
        n194 = Unbundle By Name(w752) -> ("V2 Step"=w751:dbl, "V2 Start"=w750:dbl, "Number of points"=w712:i32)
        n195 = call "4155C Split array.vi"("Number of VAR2 steps"=w712, "Y2 data in"=w725, "X data in"=w746, "Y1 data in"=w724, "Y3 data in"=w723, "error in (no error)"=w738) -> ("Array of clusters"=w739:cluster{"Y data in":dbl[], "X data in":dbl[]}[], "error out"=w700:errorcluster)  [unwired: 1 in]
        n196 = case shown="True" "Plot output curve extrema vs time" {
          tunnel: w745 -> [w808 w878]
          tunnel: w736 -> [w809 w873]
          tunnel: w727 -> [w803 w869]
          tunnel: w726 -> [w802 w868]
          tunnel: w725 -> [_ w865]
          tunnel: w724 -> [_ w863]
          tunnel: w723 -> [_ w862]
          tunnel: w722 -> [w810 w858]
          tunnel: w721 -> [w811 w857]
          tunnel: w720 -> [w806 w854]
          tunnel: w719 -> [w807 w853]
          tunnel: w718 -> [w804 w850]
          tunnel: w717 -> [w805 w849]
          tunnel: w716 -> [w800 w846]
          tunnel: w715 -> [w801 w845]
          tunnel: w714 -> [_ w838]
          tunnel: [w806 w833] -> w713
          tunnel: w712 -> [_ w832]
          tunnel: [w807 w831] -> w711
          tunnel: [w808 w830] -> w710
          tunnel: [w809 w829] -> w709
          tunnel: [w810 w828] -> w708
          tunnel: [w811 w827] -> w707
          tunnel: [w800 w826] -> w706
          tunnel: [w801 w825] -> w705
          tunnel: [w802 w824] -> w704
          tunnel: [w803 w823] -> w703
          tunnel: [w804 w822] -> w702
          tunnel: [w805 w821] -> w701
          tunnel: w700 -> [w812 w820]
          tunnel: [w812 w816] -> w699
          frame False {
          }
          frame True {
            # "Adjusts graph colors."
            # "Adjusts graph colors."
            # "Ion will be the middle element of the array. The calculation of the index is done only once, since Is, Id, and Ig have the same dimensions."
            # "abs(Ig)"
            # "abs(Is)"
            # "Y1: Is\nY2: Id\nY3: Ig"
            # "abs(Id)"
            # "Adjusts graph colors."
            # "Adjusts graph colors."
            # "Adjusts graph colors."
            n197 = Absolute Value(x=w863) -> (abs(x)=w848:dbl[])
            n198 = Absolute Value(x=w865) -> (abs(x)=w864:dbl[])
            n199 = Absolute Value(x=w862) -> (abs(x)=w851:dbl[])
            n200 = Array Size(array=w864) -> (size(s)=w872:i32)
            n201 = Divide(x=w872, y=2) -> (x/y=w815:dbl)
            n202 = Subtract(x=w815, y=1) -> (x-y=w814:dbl)
            n203 = Array Max & Min(array=w848) -> (max value=w855:dbl, min value=w856:dbl)  [unwired: 2 out]
            n204 = Array Max & Min(array=w864) -> (max value=w877:dbl, min value=w861:dbl)  [unwired: 2 out]
            n205 = Array Max & Min(array=w851) -> (max value=w860:dbl, min value=w859:dbl)  [unwired: 2 out]
            n206 = Index Array(array=w848, index=w814) -> (element=w839:dbl)
            n207 = Index Array(array=w848, index=0) -> (element=w840:dbl)
            n208 = Index Array(array=w864, index=w814) -> (element=w841:dbl)
            n209 = Index Array(array=w864, index=0) -> (element=w842:dbl)
            n210 = Index Array(array=w851, index=w814) -> (element=w844:dbl)
            n211 = Index Array(array=w851, index=0) -> (element=w843:dbl)
            n212 = local write "Ig max"(w860) -> ()
            n213 = local write "Ig min"(w859) -> ()
            n214 = local write "Is max"(w855) -> ()
            n215 = local write "Is min"(w856) -> ()
            n216 = local write "Id max"(w877) -> ()
            n217 = local write "Id min"(w861) -> ()
            n218 = Build Array (concatenate)(w854, w855) -> (w833:dbl[])
            n219 = Build Array (concatenate)(w853, w856) -> (w831:dbl[])
            n220 = local write "Is off"(w840) -> ()
            n221 = local write "Is on"(w839) -> ()
            n222 = Build Array (concatenate)(w878, w877) -> (w830:dbl[])
            n223 = Build Array (concatenate)(w873, w861) -> (w829:dbl[])
            n224 = Build Array (concatenate)(w858, w860) -> (w828:dbl[])
            n225 = Build Array (concatenate)(w857, w859) -> (w827:dbl[])
            n226 = Build Array (concatenate)(w846, w839) -> (w826:dbl[])
            n227 = Build Array (concatenate)(w845, w840) -> (w825:dbl[])
            n228 = Build Array (concatenate)(w868, w841) -> (w824:dbl[])
            n229 = Build Array (concatenate)(w869, w842) -> (w823:dbl[])
            n230 = Build Array (concatenate)(w850, w844) -> (w822:dbl[])
            n231 = Build Array (concatenate)(w849, w843) -> (w821:dbl[])
            n232 = local write "Ig off"(w843) -> ()
            n233 = local write "Ig on"(w844) -> ()
            n234 = local write "Id off"(w842) -> ()
            n235 = local write "Id on"(w841) -> ()
            n236 = control-ref of="Imax vs time"() -> (w867:refnum<vi>)
            n237 = control-ref of="Imin vs time"() -> (w866:refnum<vi>)
            n238 = control-ref of="Ion vs time"() -> (w835:refnum<vi>)
            n239 = control-ref of="Ioff vs time"() -> (w834:refnum<vi>)
            n240 = control-ref of="I vs Vg"() -> (w876:refnum<vi>)
            n241 = call "4155C Split array.vi"("Number of VAR2 steps"=w832, "Y2 data in"=w824, "X data in"=w838, "Y1 data in"=w826, "Y3 data in"=w822, "error in (no error)"=w820) -> ("Array of clusters"=w836:cluster{"Y data in":dbl[], "X data in":dbl[]}[], "error out"=w819:errorcluster)  [unwired: 1 in]
            n242 = call "4155C Split array.vi"("Number of VAR2 steps"=w832, "Y2 data in"=w823, "X data in"=w838, "Y1 data in"=w825, "Y3 data in"=w821, "error in (no error)"=w819) -> ("Array of clusters"=w837:cluster{"Y data in":dbl[], "X data in":dbl[]}[], "error out"=w818:errorcluster)  [unwired: 1 in]
            n243 = call "4155C Split array.vi"("Number of VAR2 steps"=w832, "Y2 data in"=w830, "X data in"=w838, "Y1 data in"=w833, "Y3 data in"=w828, "error in (no error)"=w818) -> ("Array of clusters"=w875:cluster{"Y data in":dbl[], "X data in":dbl[]}[], "error out"=w817:errorcluster)  [unwired: 1 in]
            n244 = call "4155C Split array.vi"("Number of VAR2 steps"=w832, "Y2 data in"=w829, "X data in"=w838, "Y1 data in"=w831, "Y3 data in"=w827, "error in (no error)"=w817) -> ("Array of clusters"=w874:cluster{"Y data in":dbl[], "X data in":dbl[]}[], "error out"=w816:errorcluster)  [unwired: 1 in]
            n245 = call "4155C Config Chart Colours.vi"("Numeric"=w832, "XY Graph 2"=w867) -> ()  [unwired: 6 in]
            n246 = call "4155C Config Chart Colours.vi"("Numeric"=w832, "XY Graph 2"=w866) -> ()  [unwired: 6 in]
            n247 = call "4155C Config Chart Colours.vi"("Numeric"=w832, "XY Graph 2"=w835) -> ()  [unwired: 6 in]
            n248 = call "4155C Config Chart Colours.vi"("Numeric"=w832, "XY Graph 2"=w834) -> ()  [unwired: 6 in]
            n249 = call "4155C Config Chart Colours.vi"("Numeric"=w832, "XY Graph 2"=w876) -> ()  [unwired: 6 in]
            n250 = local write "Imax vs time"(w875) -> ()
            n251 = local write "Imin vs time"(w874) -> ()
            n252 = local write "Ion vs time"(w836) -> ()
            n253 = local write "Ioff vs time"(w837) -> ()
          }
        }
        n254 = local write "I vs Vd"(w739) -> ()
        n255 = Open/Create/Replace File(file path (use dialog)=w791, error in=w699, operation (0:open)=w747) -> (refnum out=w734:refnum<file>, error out=w732:errorcluster)  [unwired: 3 in, 1 out]
        n256 = call "4155C Make Big 2d array.vi"("1D Var1"=w746, "1d IS"=w724, "1d ID"=w725, "1d IG"=w723, "1d SMU4"=w749, "SMU4"=w694, "VAR2 START"=w750, "Number of VAR2 steps"=w712, "VAR2 STEP"=w751, "VAR1 Name"="Vd", "Decimal places in header"=i8 1, "VAR2 Name"="Vg") -> ("Header array"=w735:string[], "Data array"=w733:dbl[][])  [unwired: 14 in]
        n257 = call "4155C Write array to file.vi"("Byte Stream File Refnum"=w734, "Header"=w735, "Data Array"=w733, "error in (no error)"=w732) -> ("dup refnum"=w731:refnum<file>, "error out"=w730:errorcluster)  [unwired: 1 in]
        n258 = Close File(refnum=w731, error in=w730) -> (error out=w786:errorcluster)  [unwired: 1 out]
      }
      frame "output-fpp" {
        n259 = Number To Decimal String(number=w896) -> (decimal integer string=w950:string)  [unwired: 1 in]
        n260 = Bundle By Name(cluster=w926, "Emergency Stop"=w953) -> (w963:T1)
        n261 = Delete From Array(array=w941, index=0 ("Index")) -> (deleted portion=w939:string, array with subset deleted=w938:string[])  [unwired: 1 in]
        n262 = VISA Write(VISA resource name=w917, write buffer=":PAGE:CHAN:MODE SWE;" ("write buffer (\"\")"), error in (no error)=w914) -> (VISA resource name out=w916:refnum<visa-resource-name>, error out=w915:errorcluster)  [unwired: 1 out]
        n263 = Concatenate Strings(w949, "-outputfpp-" ("Substring"), w950, w895, ".txt" ("Substring")) -> (w952:string)
        n264 = case shown="\"d\", Default" w939 {
          tunnel: [w964 w965] -> w937
          frame "s" {
            w964 = u16 0 items=["Single", "Double"] ("sweep mode")
          }
          frame "d", Default {
            w965 = u16 1 items=["Single", "Double"] ("sweep mode")
          }
        }
        n265 = Fract/Exp String To Number(string=w938) -> (number=w920:dbl[])  [unwired: 3 in, 1 out]
        n266 = String To Path(string=w952) -> (path=w948:path)
        n267 = Index Array(array=w920, index #1=0 ("Index")) -> (element #1=w936:dbl, element #2=w935:dbl, element #3=w934:dbl)  [unwired: 2 in]
        n268 = Delete From Array(array=w920, length=3 ("Length"), index=0 ("Index")) -> (array with subset deleted=w919:dbl[])  [unwired: 1 out]
        n269 = Bundle By Name(cluster=w928, "Gate Start"=w936, "Gate Stop"=w935, "Gate Step (linear only)"=w934, "Gate Compliance"=w946, "Range mode"=w912, "Range"=w911) -> (w962:T6)
        n270 = Index Array(array=w919, index #1=0 ("Index")) -> (element #1=w931:dbl, element #2=w930:dbl, element #3=w929:dbl)  [unwired: 2 in]
        n271 = call <vilib>:"compatOverwrite.vi"("overwrite (F)"=TRUE) -> ("overwrite?"=w900:T8)
        n272 = Bundle By Name(cluster=w927, "Drain Start"=w931, "Drain Stop"=w930, "Drain Step"=w929, "Drain Compliance"=w947, "Range mode"=w910, "Range"=w913) -> (w961:T7)
        n273 = call "4155C Output-FPP.vi"("VISA resource name in"=w916, "Gate"=w962, "Drain"=w961, "Timings"=w945, "error in (no error)"=w915, "sweep mode"=w937, "Panel controls"=w963) -> ("VD"=w905:dbl[], "Outparams"=w908:T9, "VISA Resource Name out"=w943:refnum<visa-resource-name>, "Vprobe2"=w904:dbl[], "ID"=w903:dbl[], "IG"=w902:dbl[], "Vprobe1"=w901:dbl[], "error out"=w944:errorcluster)  [unwired: 13 in]
        n274 = Unbundle By Name(w908) -> ("V2 Step"=w909:dbl, "V2 Start"=w907:dbl, "Number of points"=w906:i32)
        n275 = Open/Create/Replace File(file path (use dialog)=w948, error in=w944, operation (0:open)=w900) -> (refnum out=w958:refnum<file>, error out=w959:errorcluster)  [unwired: 3 in, 1 out]
        n276 = call "4155C Make Big 2d array FPP.vi"("1D Var1"=w905, "1d ID"=w903, "1d Vp2"=w904, "1d IG"=w902, "1d Vp1"=w901, "VAR2 START"=w907, "Number of VAR2 steps"=w906, "VAR2 STEP"=w909, "VAR1 Name"="Vd", "Decimal places in header"=i8 1, "VAR2 Name"="Vg") -> ("Header array"=w954:string[], "Data array"=w955:dbl[][])  [unwired: 15 in]
        n277 = call "4155C Write array to file.vi"("Byte Stream File Refnum"=w958, "Header"=w954, "Data Array"=w955, "error in (no error)"=w959) -> ("dup refnum"=w956:refnum<file>, "error out"=w957:errorcluster)  [unwired: 1 in]
        n278 = Close File(refnum=w956, error in=w957) -> (error out=w942:errorcluster)  [unwired: 1 out]
      }
      frame "itime" {
        n279 = Delete From Array(array=w969, index=1) -> (deleted portion=w968:string)  [unwired: 1 in, 1 out]
        n280 = Delete From Array(array=w969, index=0 ("Index")) -> (deleted portion=w997:string)  [unwired: 1 in, 1 out]
        n281 = Fract/Exp String To Number(string=w968) -> (number=w967:dbl)  [unwired: 3 in, 1 out]
        n282 = case shown="\"l\"" w997 {
          tunnel: w996 -> [w1002 w1004 w1008]
          tunnel: [w1001 w1003 w1007] -> w989
          tunnel: w967 -> [w999 _ w1006]
          frame "s" {
            w1000 = u32 0 items=["short  ", "medium  ", "long  "] ("integration time 2")
            n283 = Bundle By Name(cluster=w1002, "integration time"=w1000, "Short/Long integration time"=w999) -> (w1001:T4)
          }
          frame "m", Default {
            w1005 = u32 1 items=["short  ", "medium  ", "long  "] ("integration time 2")
            n284 = Bundle By Name(cluster=w1004, "integration time"=w1005) -> (w1003:T4)
          }
          frame "l" {
            w1009 = u32 2 items=["short  ", "medium  ", "long  "] ("integration time 2")
            n285 = Bundle By Name(cluster=w1008, "integration time"=w1009, "Short/Long integration time"=w1006) -> (w1007:T4)
          }
        }
      }
      frame "pulsed" {
        n286 = Delete From Array(array=w1038, index=0 ("Index")) -> (deleted portion=w1039:string, array with subset deleted=w1026:string[])  [unwired: 1 in]
        n287 = case shown="\"on\", Default" w1039 {
          tunnel: w1037 -> [w1049 w1052]
          tunnel: [w1048 w1051] -> w1030
          tunnel: w1026 -> [w1046 _]
          frame "on", Default {
            w1047 = u16 1 items=["Continuous", "Pulsed"] ("sweep method")
            n288 = Fract/Exp String To Number(string=w1046) -> (number=w1044:dbl[])  [unwired: 3 in, 1 out]
            n289 = Index Array(array=w1044, index #1=0 ("Index")) -> (element #1=w1043:dbl, element #2=w1042:dbl, element #3=w1041:dbl)  [unwired: 2 in]
            n290 = Bundle By Name(cluster=w1049, "sweep method"=w1047, "Pulse period"=w1043, "Base voltage"=w1042, "Pulse width"=w1041) -> (w1048:T4)
          }
          frame "off" {
            w1050 = u16 0 items=["Continuous", "Pulsed"] ("sweep method")
            n291 = Bundle By Name(cluster=w1052, "sweep method"=w1050) -> (w1051:T4)
          }
        }
      }
      frame "gaterangemode" {
        n292 = Delete From Array(array=w1079, index=0 ("Index")) -> (deleted portion=w1080:string)  [unwired: 1 in, 1 out]
        n293 = case shown="\"f\"" w1080 {
          tunnel: [w1082 w1083 w1084] -> w1069
          frame "a", Default {
            w1082 = u16 0 items=["Auto", "Limited", "Fixed"] ("Gate Range\nmode 2")
          }
          frame "f" {
            w1083 = u16 2 items=["Auto", "Limited", "Fixed"] ("Gate Range\nmode 2")
          }
          frame "l" {
            w1084 = u16 1 items=["Auto", "Limited", "Fixed"] ("Gate Range\nmode 2")
          }
        }
      }
      frame "gaterange" {
        (unwired) u8 11 items=["10fA  ", "100fA  ", "1nA  ", "10nA", "100nA", "1uA", "10uA", "100uA", "1mA", "10mA", "100mA", "1A"] ("Gate Range 2")
        n294 = Delete From Array(array=w1118, index=0 ("Index")) -> (deleted portion=w1108:string)  [unwired: 1 in, 1 out]
        n295 = Scan Value(string=w1108, format string="") -> (value=w1106:dbl)  [unwired: 1 in, 1 out]
        n296 = Logarithm Base 10(1:w1106) -> (0:w1105:dbl)
        n297 = Round To Nearest(number=w1105) -> (nearest integer value=w1104:dbl)
        n298 = Add(x=w1104, y=11.0) -> (x+y=w1102:dbl)
        n299 = To Unsigned Byte Integer(number=w1102) -> (unsigned 8bit integer=w1101:u8)
      }
      frame "drainrange" {
        (unwired) u8 11 items=["10fA  ", "100fA  ", "1nA  ", "10nA", "100nA", "1uA", "10uA", "100uA", "1mA", "10mA", "100mA", "1A"] ("Gate Range 2")
        n300 = Delete From Array(array=w1153, index=0 ("Index")) -> (deleted portion=w1144:string)  [unwired: 1 in, 1 out]
        n301 = Scan Value(string=w1144, format string="") -> (value=w1142:dbl)  [unwired: 1 in, 1 out]
        n302 = Logarithm Base 10(1:w1142) -> (0:w1141:dbl)
        n303 = Round To Nearest(number=w1141) -> (nearest integer value=w1140:dbl)
        n304 = Add(x=w1140, y=11.0) -> (x+y=w1138:dbl)
        n305 = To Unsigned Byte Integer(number=w1138) -> (unsigned 8bit integer=w1137:u8)
      }
      frame "drainrangemode" {
        n306 = Delete From Array(array=w1181, index=0 ("Index")) -> (deleted portion=w1182:string)  [unwired: 1 in, 1 out]
        n307 = case shown="\"f\"" w1182 {
          tunnel: [w1184 w1185 w1186] -> w1171
          frame "a", Default {
            w1184 = u16 0 items=["Auto", "Limited", "Fixed"] ("Gate Range\nmode 2")
          }
          frame "f" {
            w1185 = u16 2 items=["Auto", "Limited", "Fixed"] ("Gate Range\nmode 2")
          }
          frame "l" {
            w1186 = u16 1 items=["Auto", "Limited", "Fixed"] ("Gate Range\nmode 2")
          }
        }
      }
      frame "Error", Default {
      }
      frame "logfile" {
        n308 = Number To Decimal String(number=w1229) -> (decimal integer string=w1264:string)  [unwired: 1 in]
        n309 = Concatenate Strings(w1263, "logfile" ("Substring"), w1264, w1227, ".txt" ("Substring")) -> (w1261:string)
        n310 = String To Path(string=w1261) -> (path=w1234:path)
        n311 = Unbundle(w1260) -> ("integration time"=w1259:u32, "Short/Long integration time"=w1258:dbl, "hold time (sec)"=w1257:dbl, "delay time (sec)"=w1256:dbl, "Step Time (0 disables)"=w1255:dbl, "sweep method"=w1254:u16, "Pulse period"=w1253:dbl, "Base voltage"=w1252:dbl, "Pulse width"=w1251:dbl)
        n312 = Build Array(w1259, w1258, w1257, w1256, w1255, w1254, w1253, w1252, w1251, w1245, w1246, w1247, w1248, w1249, w1250) -> (w1238:dbl[])
        n313 = Insert Into Array(array=dbl[][] [] ("Input Array"), new element=w1238) -> (w1237:dbl[][])  [unwired: 2 in]
        n314 = call <vilib>:"compatOverwrite.vi"("overwrite (F)"=TRUE) -> ("overwrite?"=w1232:T8)
        n315 = Open/Create/Replace File(file path (use dialog)=w1234, error in=w1236, operation (0:open)=w1232) -> (refnum out=w1242:refnum<file>, error out=w1241:errorcluster)  [unwired: 3 in, 1 out]
        n316 = call "4155C Write array to file.vi"("Byte Stream File Refnum"=w1242, "Header"=string[] ["Int Time", "Short/Long Itime", "Hold time", "Delay time", "Step time", "Sweep method", "Pulse period", "Base Voltage", "Pulse width", "Drain compliance", "Gate compliance", "Gate range mode", "Gate range", "S/D range mode", "S/D range"], "Data Array"=w1237, "error in (no error)"=w1241) -> ("dup refnum"=w1244:refnum<file>, "error out"=w1243:errorcluster)  [unwired: 1 in]
        n317 = Close File(refnum=w1244, error in=w1243) -> (error out=w1235:errorcluster)  [unwired: 1 out]
      }
      frame "sample" {
        n318 = Number To Decimal String(number=w1282) -> (decimal integer string=w1330:string)  [unwired: 1 in]
        n319 = Fract/Exp String To Number(string=w1327) -> (number=w1288:dbl[])  [unwired: 3 in, 1 out]
        n320 = Concatenate Strings(w1305, "-sample-" ("Substring"), w1330, w1280, ".txt" ("Substring")) -> (w1328:string)
        n321 = Index Array(array=w1288, index=0 ("Index")) -> (element=w1325:dbl)
        n322 = String To Path(string=w1328) -> (path=w1309:path)
        n323 = Index Array(array=w1288, index=2 ("Index")) -> (element=w1321:dbl)
        n324 = Index Array(array=w1288, index=3 ("Index")) -> (element=w1290:dbl)
        n325 = Index Array(array=w1288, index=4 ("Index")) -> (element=w1287:dbl)
        n326 = call "4155C Config Sampling Measurements.vi"("Sampling interval"=w1287, "Sample time"=w1290, "Display on/off"=TRUE, "Timings"=w1296, "Num Points"=w1321, "error in (no error)"=w1332, "Drain Compliance"=w1331, "Gate Compliance"=w1306, "VISA session"=w1333) -> ("error out"=w1334:errorcluster, "dup VISA resource name"=w1335:refnum<visa-resource-name>)  [unwired: 1 in]
        n327 = Index Array(array=w1288, index=1 ("Index")) -> (element=w1322:dbl)
        n328 = call "4155C Take Sample.vi"("Emergency Stop"=w1302, "error in (no error)"=w1334, "Vd"=w1322, "Vg"=w1325, "VISA resource name in"=w1335) -> ("error out"=w1300:errorcluster, "Id"=w1337:dbl[], "Ig"=w1311:dbl[], "VISA Resource Name out"=w1298:refnum<visa-resource-name>, "Is"=w1336:dbl[], "Time"=w1315:dbl[])  [unwired: 1 in]
        n329 = Insert Into Array(array=dbl[][] [] ("Input Array"), new element=w1315) -> (w1314:dbl[][])  [unwired: 2 in]
        n330 = Insert Into Array(array=w1314, new element=w1311) -> (w1313:dbl[][])  [unwired: 2 in]
        n331 = Insert Into Array(array=w1313, new element=w1337) -> (w1312:dbl[][])  [unwired: 2 in]
        n332 = VISA Write(VISA resource name=w1298, write buffer=":DISP ON" ("write buffer (\"\")"), error in (no error)=w1300) -> (VISA resource name out=w1297:refnum<visa-resource-name>, error out=w1299:errorcluster)  [unwired: 1 out]
        n333 = Insert Into Array(array=w1312, new element=w1336) -> (w1304:dbl[][])  [unwired: 2 in]
        n334 = Transpose 2D Array(2D array=w1304) -> (transposed array=w1303:dbl[][])
        n335 = call <vilib>:"compatOverwrite.vi"("overwrite (F)"=TRUE) -> ("overwrite?"=w1285:T8)
        n336 = Open/Create/Replace File(file path (use dialog)=w1309, error in=w1299, operation (0:open)=w1285) -> (refnum out=w1318:refnum<file>, error out=w1317:errorcluster)  [unwired: 3 in, 1 out]
        n337 = call "4155C Write array to file.vi"("Byte Stream File Refnum"=w1318, "Header"=string[] ["Time /s", "Ig /A", "Id /A", "Is /A"], "Data Array"=w1303, "error in (no error)"=w1317) -> ("dup refnum"=w1320:refnum<file>, "error out"=w1319:errorcluster)  [unwired: 1 in]
        n338 = Close File(refnum=w1320, error in=w1319) -> (error out=w1307:errorcluster)  [unwired: 1 out]
      }
      frame "samplei" {
        n339 = Number To Decimal String(number=w1354) -> (decimal integer string=w1405:string)  [unwired: 1 in]
        n340 = Concatenate Strings(w1384, "-samplei-" ("Substring"), w1405, w1353, ".txt" ("Substring")) -> (w1403:string)
        n341 = Fract/Exp String To Number(string=w1402) -> (number=w1369:dbl[])  [unwired: 3 in, 1 out]
        n342 = String To Path(string=w1403) -> (path=w1387:path)
        n343 = Index Array(array=w1369, index=4 ("Index")) -> (element=w1363:dbl)
        n344 = Index Array(array=w1369, index=3 ("Index")) -> (element=w1364:dbl)
        n345 = Index Array(array=w1369, index=1 ("Index")) -> (element=w1366:dbl)
        n346 = Index Array(array=w1369, index=0 ("Index")) -> (element=w1367:dbl)
        n347 = Index Array(array=w1369, index=2 ("Index")) -> (element=w1365:dbl)
        n348 = call "4155C Config SamplingI Measurements.vi"("Sample time"=w1365, "Display on/off"=TRUE, "Timings"=w1376, "Num Points"=w1366, "error in (no error)"=w1407, "Sampling interval"=w1364, "VISA session"=w1408) -> ("error out"=w1409:errorcluster, "dup VISA resource name"=w1410:refnum<visa-resource-name>)  [unwired: 3 in]
        n349 = call "4155C Take SampleI.vi"("Emergency Stop"=w1381, "error in (no error)"=w1409, "Idg 2"=w1367, "Vdg compliance 2"=w1363, "VISA resource name in"=w1410) -> ("error out"=w1379:errorcluster, "Idg"=w1412:dbl[], "Vdg"=w1389:dbl[], "VISA Resource Name out"=w1377:refnum<visa-resource-name>, "Is"=w1411:dbl[], "Time"=w1393:dbl[])  [unwired: 1 in]
        n350 = Insert Into Array(array=dbl[][] [] ("Input Array"), new element=w1393) -> (w1392:dbl[][])  [unwired: 2 in]
        n351 = Insert Into Array(array=w1392, new element=w1389) -> (w1391:dbl[][])  [unwired: 2 in]
        n352 = Insert Into Array(array=w1391, new element=w1412) -> (w1390:dbl[][])  [unwired: 2 in]
        n353 = VISA Write(VISA resource name=w1377, write buffer=":DISP ON" ("write buffer (\"\")"), error in (no error)=w1379) -> (VISA resource name out=w1362:refnum<visa-resource-name>, error out=w1378:errorcluster)  [unwired: 1 out]
        n354 = Insert Into Array(array=w1390, new element=w1411) -> (w1383:dbl[][])  [unwired: 2 in]
        n355 = call <vilib>:"compatOverwrite.vi"("overwrite (F)"=TRUE) -> ("overwrite?"=w1357:T8)
        n356 = Open/Create/Replace File(file path (use dialog)=w1387, error in=w1378, operation (0:open)=w1357) -> (refnum out=w1396:refnum<file>, error out=w1395:errorcluster)  [unwired: 3 in, 1 out]
        n357 = Transpose 2D Array(2D array=w1383) -> (transposed array=w1382:dbl[][])
        n358 = call "4155C Write array to file.vi"("Byte Stream File Refnum"=w1396, "Header"=string[] ["Time /s", "Vdg /V", "Idg /A", "Is /A"], "Data Array"=w1382, "error in (no error)"=w1395) -> ("dup refnum"=w1398:refnum<file>, "error out"=w1397:errorcluster)  [unwired: 1 in]
        n359 = Close File(refnum=w1398, error in=w1397) -> (error out=w1360:errorcluster)  [unwired: 1 out]
        n360 = VISA Write(VISA resource name=w1362, write buffer=";:PAGE:SCON:STAN OFF;:PAGE:CHAN:VSU2:DIS;" ("write buffer (\"\")"), error in (no error)=w1360) -> (VISA resource name out=w1358:refnum<visa-resource-name>, error out=w1359:errorcluster)  [unwired: 1 out]
      }
      frame "#" {
        n361 = VISA Write(VISA resource name=w1433, write buffer=":DISP ON" ("write buffer (\"\")"), error in (no error)=w1432) -> (VISA resource name out=w1431:refnum<visa-resource-name>, error out=w1430:errorcluster)  [unwired: 1 out]
      }
      frame "stressV" {
        n362 = Number To Decimal String(number=w1457) -> (decimal integer string=w1498:string)  [unwired: 1 in]
        n363 = Concatenate Strings(w1482, "-stressV-" ("Substring"), w1498, w1456, ".txt" ("Substring")) -> (w1496:string)
        n364 = Fract/Exp String To Number(string=w1495) -> (number=w1468:dbl[])  [unwired: 3 in, 1 out]
        n365 = String To Path(string=w1496) -> (path=w1486:path)
        n366 = Index Array(array=w1468, index=3 ("Index")) -> (element=w1465:dbl)
        n367 = Index Array(array=w1468, index=1 ("Index")) -> (element=w1463:dbl)
        n368 = Index Array(array=w1468, index=0 ("Index")) -> (element=w1462:dbl)
        n369 = Index Array(array=w1468, index=4 ("Index")) -> (element=w1467:dbl)
        n370 = Index Array(array=w1468, index=2 ("Index")) -> (element=w1464:dbl)
        n371 = call "4155C Config V Stress.vi"("VISA session"=w1501, "ID compliance"=w1465, "VD"=w1463, "VG"=w1462, "IG compliance"=w1464, "error in (no error)"=w1500, "Display on/off"=TRUE) -> ("dup VISA resource name"=w1503:refnum<visa-resource-name>, "error out"=w1502:errorcluster)
        n372 = call "4155C Apply Stress.vi"("error in (no error)"=w1502, "Duration"=w1467, "Emergency Stop"=w1481, "VISA resource name in"=w1503) -> ("error out"=w1479:errorcluster, "VISA Resource Name out"=w1477:refnum<visa-resource-name>)
        n373 = VISA Write(VISA resource name=w1477, write buffer=":DISP ON" ("write buffer (\"\")"), error in (no error)=w1479) -> (VISA resource name out=w1476:refnum<visa-resource-name>, error out=w1478:errorcluster)  [unwired: 1 out]
        n374 = call <vilib>:"compatOverwrite.vi"("overwrite (F)"=TRUE) -> ("overwrite?"=w1461:T8)
        n375 = Open/Create/Replace File(file path (use dialog)=w1486, error in=w1478, operation (0:open)=w1461) -> (refnum out=w1489:refnum<file>, error out=w1488:errorcluster)  [unwired: 3 in, 1 out]
        n376 = call "4155C Write array to file.vi"("Byte Stream File Refnum"=w1489, "Header"=string[] ["V stress completed successfully", ""], "error in (no error)"=w1488) -> ("dup refnum"=w1491:refnum<file>, "error out"=w1490:errorcluster)  [unwired: 2 in]
        n377 = Close File(refnum=w1491, error in=w1490) -> (error out=w1484:errorcluster)  [unwired: 1 out]
      }
      frame "stressI" {
        n378 = Number To Decimal String(number=w1519) -> (decimal integer string=w1556:string)  [unwired: 1 in]
        n379 = Concatenate Strings(w1540, "-stressI-" ("Substring"), w1556, w1518, ".txt" ("Substring")) -> (w1554:string)
        n380 = Fract/Exp String To Number(string=w1553) -> (number=w1528:dbl[])  [unwired: 3 in, 1 out]
        n381 = Index Array(array=w1528, index=1 ("Index")) -> (element=w1524:dbl)
        n382 = Index Array(array=w1528, index=0 ("Index")) -> (element=w1525:dbl)
        n383 = call "4155C Config I Stress.vi"("VISA session"=w1559, "IDG"=w1525, "VDG compliance"=w1524, "error in (no error)"=w1558, "Display on/off"=TRUE) -> ("dup VISA resource name"=w1561:refnum<visa-resource-name>, "error out"=w1560:errorcluster)
        n384 = Index Array(array=w1528, index=2 ("Index")) -> (element=w1526:dbl)
        n385 = String To Path(string=w1554) -> (path=w1544:path)
        n386 = call "4155C Apply Stress.vi"("error in (no error)"=w1560, "Duration"=w1526, "Emergency Stop"=w1539, "VISA resource name in"=w1561) -> ("error out"=w1537:errorcluster, "VISA Resource Name out"=w1535:refnum<visa-resource-name>)
        n387 = VISA Write(VISA resource name=w1535, write buffer=":DISP ON" ("write buffer (\"\")"), error in (no error)=w1537) -> (VISA resource name out=w1534:refnum<visa-resource-name>, error out=w1536:errorcluster)  [unwired: 1 out]
        n388 = call <vilib>:"compatOverwrite.vi"("overwrite (F)"=TRUE) -> ("overwrite?"=w1523:T8)
        n389 = Open/Create/Replace File(file path (use dialog)=w1544, error in=w1536, operation (0:open)=w1523) -> (refnum out=w1547:refnum<file>, error out=w1546:errorcluster)  [unwired: 3 in, 1 out]
        n390 = call "4155C Write array to file.vi"("Byte Stream File Refnum"=w1547, "Header"=string[] ["I stress completed successfully", ""], "error in (no error)"=w1546) -> ("dup refnum"=w1549:refnum<file>, "error out"=w1548:errorcluster)  [unwired: 2 in]
        n391 = Close File(refnum=w1549, error in=w1548) -> (error out=w1542:errorcluster)  [unwired: 1 out]
      }
      frame "vsu2pulse" {
        n392 = Number To Decimal String(number=w1577) -> (decimal integer string=w1612:string)  [unwired: 1 in]
        n393 = Concatenate Strings(w1597, "-vsu2-" ("Substring"), w1612, w1576, ".txt" ("Substring")) -> (w1610:string)
        n394 = Fract/Exp String To Number(string=w1609) -> (number=w1585:dbl[])  [unwired: 3 in, 1 out]
        n395 = String To Path(string=w1610) -> (path=w1601:path)
        n396 = Index Array(array=w1585, index=1 ("Index")) -> (element=w1584:dbl)
        n397 = Index Array(array=w1585, index=0 ("Index")) -> (element=w1582:dbl)
        n398 = call "4155C Config VSU2 Stress.vi"("error in (no error)"=w1614, "VSU2"=w1582, "Display on/off"=TRUE, "VISA session"=w1615) -> ("error out"=w1616:errorcluster, "dup VISA resource name"=w1617:refnum<visa-resource-name>)
        n399 = call "4155C Apply Stress.vi"("error in (no error)"=w1616, "Duration"=w1584, "Emergency Stop"=w1596, "VISA resource name in"=w1617) -> ("error out"=w1594:errorcluster, "VISA Resource Name out"=w1592:refnum<visa-resource-name>)
        n400 = VISA Write(VISA resource name=w1592, write buffer=":DISP ON" ("write buffer (\"\")"), error in (no error)=w1594) -> (VISA resource name out=w1591:refnum<visa-resource-name>, error out=w1593:errorcluster)  [unwired: 1 out]
        n401 = call <vilib>:"compatOverwrite.vi"("overwrite (F)"=TRUE) -> ("overwrite?"=w1581:T8)
        n402 = Open/Create/Replace File(file path (use dialog)=w1601, error in=w1593, operation (0:open)=w1581) -> (refnum out=w1604:refnum<file>, error out=w1603:errorcluster)  [unwired: 3 in, 1 out]
        n403 = call "4155C Write array to file.vi"("Byte Stream File Refnum"=w1604, "Header"=string[] ["VSU2 pulse completed successfully", ""], "error in (no error)"=w1603) -> ("dup refnum"=w1606:refnum<file>, "error out"=w1605:errorcluster)  [unwired: 2 in]
        n404 = Close File(refnum=w1606, error in=w1605) -> (error out=w1599:errorcluster)  [unwired: 1 out]
      }
      frame "sample-fpp" {
        w1644 = string[] ["Time /s", "Id VgVd /A", "Ig VgVd /A", "Vp1 VgVd /V", "Vp2 VgVd /V"] ("Header")
        w1648 = "%d" ("format string")
        n405 = Number To Decimal String(number=w1633) -> (decimal integer string=w1696:string)  [unwired: 1 in]
        n406 = Fract/Exp String To Number(string=w1693) -> (number=w1681:dbl[])  [unwired: 3 in, 1 out]
        n407 = Concatenate Strings(w1687, "-samplefpp-" ("Substring"), w1696, w1632, ".txt" ("Substring")) -> (w1694:string)
        n408 = String To Path(string=w1694) -> (path=w1656:path)
        n409 = Index Array(array=w1681, index=0 ("Index")) -> (element=w1642:dbl)
        n410 = Index Array(array=w1681, index=1 ("Index")) -> (element=w1641:dbl)
        n411 = Index Array(array=w1681, index=2 ("Index")) -> (element=w1689:dbl)
        n412 = Index Array(array=w1681, index=3 ("Index")) -> (element=w1679:dbl)
        n413 = call "4155C Config Sampling Measurements FPP.vi"("VISA session"=w1699, "Num Points"=w1689, "Vg"=w1642, "Display on/off"=TRUE, "Gate Compliance"=w1688, "Drain Compliance"=w1697, "Standby"="Standby", "error in (no error)"=w1698, "Timings"=w1686, "Vd"=w1641, "Sample time"=w1679) -> ("dup VISA resource name"=w1658:refnum<visa-resource-name>, "error out"=w1657:errorcluster)  [unwired: 3 in]
        n414 = Number To Decimal String(number=w1642) -> (decimal integer string=w1668:string)  [unwired: 1 in]
        n415 = call "4155C Take Sample FPP.vi"("VISA resource name in"=w1658, "error in (no error)"=w1657, "Emergency Stop"=w1659) -> ("Time"=w1663:dbl[], "Vp1"=w1673:dbl[], "VISA Resource Name out"=w1639:refnum<visa-resource-name>, "Ig"=w1661:dbl[], "Id"=w1662:dbl[], "Vp2"=w1671:dbl[], "error out"=w1660:errorcluster)  [unwired: 10 in]
        n416 = Insert Into Array(array=dbl[][] [] ("Input Array"), new element=w1663) -> (w1677:dbl[][])  [unwired: 2 in]
        n417 = Number To Decimal String(number=w1641) -> (decimal integer string=w1666:string)  [unwired: 1 in]
        n418 = Insert Into Array(array=w1677, new element=w1662) -> (w1676:dbl[][])  [unwired: 2 in]
        n419 = Concatenate Strings("(Vg = " ("Substring"), w1668, "V, Vd = " ("Substring"), w1666, "V)" ("Substring")) -> (w1664:string)
        n420 = Insert Into Array(array=w1676, new element=w1661) -> (w1675:dbl[][])  [unwired: 2 in]
        n421 = Insert Into Array(array=w1675, new element=w1673) -> (w1672:dbl[][])  [unwired: 2 in]
        n422 = Insert Into Array(array=w1672, new element=w1671) -> (w1640:dbl[][])  [unwired: 2 in]
        n423 = Transpose 2D Array(2D array=w1640) -> (transposed array=w1670:dbl[][])
        n424 = call <vilib>:"compatOverwrite.vi"("overwrite (F)"=TRUE) -> ("overwrite?"=w1637:T8)
        n425 = Open/Create/Replace File(file path (use dialog)=w1656, error in=w1660, operation (0:open)=w1637) -> (refnum out=w1653:refnum<file>, error out=w1654:errorcluster)  [unwired: 3 in, 1 out]
        n426 = Array To Spreadsheet String(array=w1644, 3:w1648) -> (spreadsheet string=w1650:string)  [unwired: 1 in]
        n427 = Search and Replace String(replace all?=TRUE ("replace all? (F)"), input string=w1650, search string="VgVd", replace string=w1664) -> (result string=w1646:string)  [unwired: 4 in, 3 out]
        n428 = Spreadsheet String To Array(format string=w1648, spreadsheet string=w1646, array type (2D Dbl)=w1644) -> (array=w1645:string[])  [unwired: 1 in]
        n429 = call "4155C Write array to file.vi"("Byte Stream File Refnum"=w1653, "Header"=w1645, "Data Array"=w1670, "error in (no error)"=w1654) -> ("dup refnum"=w1651:refnum<file>, "error out"=w1652:errorcluster)  [unwired: 1 in]
        n430 = Close File(refnum=w1651, error in=w1652) -> (error out=w1638:errorcluster)  [unwired: 1 out]
      }
      frame "resample-fpp" {
        w1728 = string[] ["Time /s", "Id VgVd /A", "Ig VgVd /A", "Vp1 VgVd /V", "Vp2 VgVd /V"] ("Header")
        w1732 = "%d" ("format string")
        n431 = Number To Decimal String(number=w1714) -> (decimal integer string=w1772:string)  [unwired: 1 in]
        n432 = Fract/Exp String To Number(string=w1769) -> (number=w1721:dbl[])  [unwired: 3 in, 1 out]
        n433 = Concatenate Strings(w1765, "-resamplefpp-" ("Substring"), w1772, w1715, ".txt" ("Substring")) -> (w1770:string)
        n434 = String To Path(string=w1770) -> (path=w1740:path)
        n435 = Index Array(array=w1721, index=0 ("Index")) -> (element=w1727:dbl)
        n436 = Index Array(array=w1721, index=1 ("Index")) -> (element=w1726:dbl)
        n437 = Number To Decimal String(number=w1727) -> (decimal integer string=w1750:string)  [unwired: 1 in]
        n438 = call "4155C Take Sample FPP.vi"("VISA resource name in"=w1723, "error in (no error)"=w1722, "Emergency Stop"=w1741) -> ("Time"=w1745:dbl[], "Vp1"=w1755:dbl[], "VISA Resource Name out"=w1725:refnum<visa-resource-name>, "Ig"=w1743:dbl[], "Id"=w1744:dbl[], "Vp2"=w1753:dbl[], "error out"=w1742:errorcluster)  [unwired: 10 in]
        n439 = Insert Into Array(array=dbl[][] [] ("Input Array"), new element=w1745) -> (w1759:dbl[][])  [unwired: 2 in]
        n440 = Number To Decimal String(number=w1726) -> (decimal integer string=w1748:string)  [unwired: 1 in]
        n441 = Insert Into Array(array=w1759, new element=w1744) -> (w1758:dbl[][])  [unwired: 2 in]
        n442 = Concatenate Strings("(Vg = " ("Substring"), w1750, "V, Vd = " ("Substring"), w1748, "V)" ("Substring")) -> (w1746:string)
        n443 = Insert Into Array(array=w1758, new element=w1743) -> (w1757:dbl[][])  [unwired: 2 in]
        n444 = Insert Into Array(array=w1757, new element=w1755) -> (w1754:dbl[][])  [unwired: 2 in]
        n445 = Insert Into Array(array=w1754, new element=w1753) -> (w1720:dbl[][])  [unwired: 2 in]
        n446 = call <vilib>:"compatOverwrite.vi"("overwrite (F)"=TRUE) -> ("overwrite?"=w1719:T8)
        n447 = Open/Create/Replace File(file path (use dialog)=w1740, error in=w1742, operation (0:open)=w1719) -> (refnum out=w1737:refnum<file>, error out=w1738:errorcluster)  [unwired: 3 in, 1 out]
        n448 = Array To Spreadsheet String(array=w1728, 3:w1732) -> (spreadsheet string=w1734:string)  [unwired: 1 in]
        n449 = Transpose 2D Array(2D array=w1720) -> (transposed array=w1752:dbl[][])
        n450 = Search and Replace String(replace all?=TRUE ("replace all? (F)"), input string=w1734, search string="VgVd", replace string=w1746) -> (result string=w1730:string)  [unwired: 4 in, 3 out]
        n451 = Spreadsheet String To Array(format string=w1732, spreadsheet string=w1730, array type (2D Dbl)=w1728) -> (array=w1729:string[])  [unwired: 1 in]
        n452 = call "4155C Write array to file.vi"("Byte Stream File Refnum"=w1737, "Header"=w1729, "Data Array"=w1752, "error in (no error)"=w1738) -> ("dup refnum"=w1735:refnum<file>, "error out"=w1736:errorcluster)  [unwired: 1 in]
        n453 = Close File(refnum=w1735, error in=w1736) -> (error out=w1724:errorcluster)  [unwired: 1 out]
      }
      frame "serial" {
        n454 = local read "Termination char\n(0xA = '\\n' = LF)\n(0xD = '\\r' = CR)"() -> (w1795:u8)
        n455 = local read "Enable Termination\nChar (T)"() -> (w1796:bool)
        n456 = Index Array(array=w1803, index=0 ("Index")) -> (element=w1802:string)
        n457 = local read "parity"() -> (w1786:u16)
        n458 = local read "Delay before read (ms)"() -> (w1797:u32)
        n459 = local read "byte count"() -> (w1794:u32)
        n460 = local read "Timeout (ms)"() -> (w1793:u32)
        n461 = local read "VISA resource name"() -> (w1790:refnum<visa-resource-name>)
        n462 = local read "baud rate"() -> (w1789:u32)
        n463 = local read "Serial End Mode for Reads"() -> (w1788:u16)
        n464 = local read "data bits"() -> (w1787:u16)
        n465 = local read "stop bits"() -> (w1792:u16)
        n466 = local read "flow control"() -> (w1791:u16)
        n467 = call "Serial write and read v0.5.vi"("Delay before read (ms)"=w1797, "Termination char\n(0xA = '\\n' = LF)\n(0xD = '\\r' = CR)"=w1795, "Enable Termination\nChar (T)"=w1796, "parity"=w1786, "stop bits"=w1792, "string to write"=w1802, "flow control"=w1791, "byte count"=w1794, "Serial Settings:Serial End Mode for Reads"=w1788, "Timeout (ms)"=w1793, "error in (no error)"=w1808, "VISA resource name"=w1790, "baud rate"=w1789, "data bits"=w1787) -> ("Serial port output"=w1798:string, "error out"=w1807:errorcluster)
        n468 = Build Array (concatenate)(w1798, w1799) -> (w1800:string[])
      }
    }
    n469 = local read "Time Units"() -> (w66:u16)
    n470 = case shown="0" w66 {
      tunnel: ["Time (Seconds)" ("element") "Time (Minutes)" ("element") "Time (Hours)" ("element")] -> w106
      frame 0 {
      }
      frame 1, Default {
      }
      frame 2 {
      }
    }
    n471 = Build Array(w119, w74, w84, w83, w82, w81, w80, w79, w78, w77, w76, w75, w73) -> (w141:dbl[][])
    n472 = Transpose 2D Array(2D array=w141) -> (transposed array=w140:dbl[][])
    n473 = Concatenate Strings(w71, "-Imax_Imin_Ion_Ioff_vs_time.txt" ("Suffix (Imax,Imin,Ion,Ioff)")) -> (w151:string)
    n474 = Build Array(w106, "Is max (A)" ("VAR2 Name"), "Is min (A)" ("VAR2 Name"), "Id max (A)" ("VAR2 Name"), "Id min (A)" ("VAR2 Name"), "Ig max (A)" ("VAR2 Name"), "Ig min (A)" ("VAR2 Name"), "Is on (A)" ("VAR2 Name"), "Is off (A)" ("VAR2 Name"), "Id on (A)" ("VAR2 Name"), "Id off (A)" ("VAR2 Name"), "Ig on (A)" ("VAR2 Name"), "Ig off (A)" ("VAR2 Name")) -> (w146:string[])
    n475 = Array To Spreadsheet String(array=w140, 3:"%e" ("format string")) -> (spreadsheet string=w144:string)  [unwired: 1 in]
    n476 = Array To Spreadsheet String(array=w146, 3:"" ("format string")) -> (spreadsheet string=w145:string)  [unwired: 1 in]
    n477 = String To Path(string=w151) -> (path=w150:path)
    n478 = Build Array(w145, w144) -> (w143:string[])
    n479 = Write to Text File(file (use dialog)=w150, text=w143, error in=w117) -> (refnum out=w152:refnum<file>, error out=w142:errorcluster)  [unwired: 1 in, 1 out]
    n480 = Close File(refnum=w152, error in=w142) -> (error out=w70:errorcluster)  [unwired: 1 out]
    n481 = Concatenate Strings(w71, "-serial_port_output.txt" ("Suffix (serial port log)")) -> (w121:string)
    n482 = String To Path(string=w121) -> (path=w120:path)
    n483 = Build Array(w106, "Serial port input" ("VAR2 Name"), "Serial port output: ") -> (w110:string[])
    n484 = Array To Spreadsheet String(array=w114, 3:"" ("format string")) -> (spreadsheet string=w107:string)  [unwired: 1 in]
    n485 = Array To Spreadsheet String(array=w110, 3:"" ("format string")) -> (spreadsheet string=w108:string)  [unwired: 1 in]
    n486 = Build Array(w108, w107) -> (w109:string[])
    n487 = Array To Spreadsheet String(array=w113, 3:"" ("format string")) -> (spreadsheet string=w126:string)  [unwired: 1 in]
    n488 = Write to Text File(file (use dialog)=w120, text=w109, error in=w70) -> (refnum out=w122:refnum<file>, error out=w123:errorcluster)  [unwired: 1 in, 1 out]
    n489 = Close File(refnum=w122, error in=w123) -> (error out=w68:errorcluster)  [unwired: 1 out]
    n490 = local write "Serial port data"(w126) -> ()
  }
  "error out" <- w27
  "Timings Indicator" <- w18
  "SMU4 Indicator" <- w1
  "Is max" <- w12
  "Id max" <- w12
  "Ig max" <- w12
  "Imax vs time" <- w8
  "I vs Vg" <- w8
  "Imin vs time" <- w8
  "I vs Vd" <- w8
  "Serial port data" <- "" ("Serial port data")
  "Is min" <- w11
  "Id min" <- w11
  "Ig min" <- w11
  "Ion vs time" <- w8
  "Ioff vs time" <- w8
  "Is on" <- w10
  "Id on" <- w10
  "Ig on" <- w10
  "Is off" <- w9
  "Id off" <- w9
  "Ig off" <- w9
